vi "运维调试_氨氮总磷.vi"() -> ()   [LabVIEW 2016, in "氨氮总磷.lvlib"]
uses:
  <vilib>/Utility/miscctls.llb/LVPointTypeDef.ctl
  <vilib>/Utility/config.llb/NI_LVConfig.lvlib
panel:
  in  "氨氮自动测试量程配置":T1={"水样测试量程模式"=enum."AUTO", "空白核查量程模式"=enum."AUTO", "跨度核查量程模式"=enum."AUTO"}
  in  "总磷自动测试量程配置":T1={"水样测试量程模式"=enum."AUTO", "空白核查量程模式"=enum."AUTO", "跨度核查量程模式"=enum."AUTO"}
  in  "质控参数设置":bool
  out "字符串":string
  out "ADC":sgl
  out "温度2":sgl
  out "温度1":sgl
  out "总磷测量数据":T2(xcontrol)
  out "固件版本号":string
  in  "数组":string[](array[string])
  in  "备用系数写入":bool
  in  "备用系数读取":bool
  in  "备用系数":T3
  in  "量程切换阈值写入":bool
  in  "量程切换阈值读取":bool
  in  "量程切换阈值":cluster{"阈值":dbl, "标液浓度":dbl}
  in  "参数下拉列表":enum16{"氨氮", "总磷"}(ring)
  in  "量程下拉列表":enum16{"低量程", "高量程"}(ring)
  in  "测量模式下拉列表":enum16{"水样测量", "空白核查", "标样核查", "盲样测试", "加标回收"}(ring)
  in  "公式":cluster{"X^2":dbl, "X":dbl, "b":dbl}
  in  "写公式":bool
  in  "读公式":bool
  in  "精度":dbl=4.0
  in  "样品5 F0":dbl
  in  "样品5 F1":dbl
  in  "样品4 F1":dbl
  in  "样品4 F0":dbl
  in  "样品3 F0":dbl
  in  "样品3 F1":dbl
  in  "样品2 F0":dbl
  in  "样品2 F1":dbl
  in  "样品1 F1":dbl
  in  "样品1 F0":dbl
  in  "method":u16(ring) items=["最小二乘", "最小绝对残差", "Bisquare"]
  in  "模型":enum32{"线性", "多项式"}(ring)
  out "r^2":dbl format="%.7g"
  out "拟合公式":string
  in  "样品2启用":bool
  in  "样品5启用":bool
  in  "样品4启用":bool
  in  "样品3启用":bool
  in  "样品1启用":bool
  in  "标液浓度5":dbl
  in  "测量吸光度5":dbl
  in  "标液浓度4":dbl
  in  "测量吸光度4":dbl
  in  "标液浓度3":dbl
  in  "测量吸光度3":dbl
  in  "标液浓度2":dbl
  in  "测量吸光度2":dbl
  in  "测量吸光度1":dbl
  in  "标液浓度1":dbl
  out "XY图":cluster{"X Values":dbl[], "Y Values":dbl[]}[](graph)
  in  "返回":bool
  in  "设置":bool
  out "序列号":string="序列号"
  out "氨氮测量数据":T2(xcontrol)
  out "集成报警信息":string
  out "定时启动":bool
  out "总磷总氮运行状态":T4(xcontrol)
  in  "停止":bool
  in  "手动启动":bool
  in  "单步测试":bool
  in  "总磷氨氮调试":u16[](xcontrol)
  out "F3":sgl format="%#.6f"
  out "F2":sgl format="%#.6f"
  out "F1":sgl format="%#.6f"
  out "F0":sgl format="%#.6f"
  out "多列列表框":i32(listbox)
  # "参数设置"
  # "标液浓度"
  # "F0"
  # "F1"
  # "吸光值显示"
  # "样品一"
  # "辅\n助\n计\n算\n区"
  # "样品二"
  # "样品三"
  # "样品四"
  # "样品五"
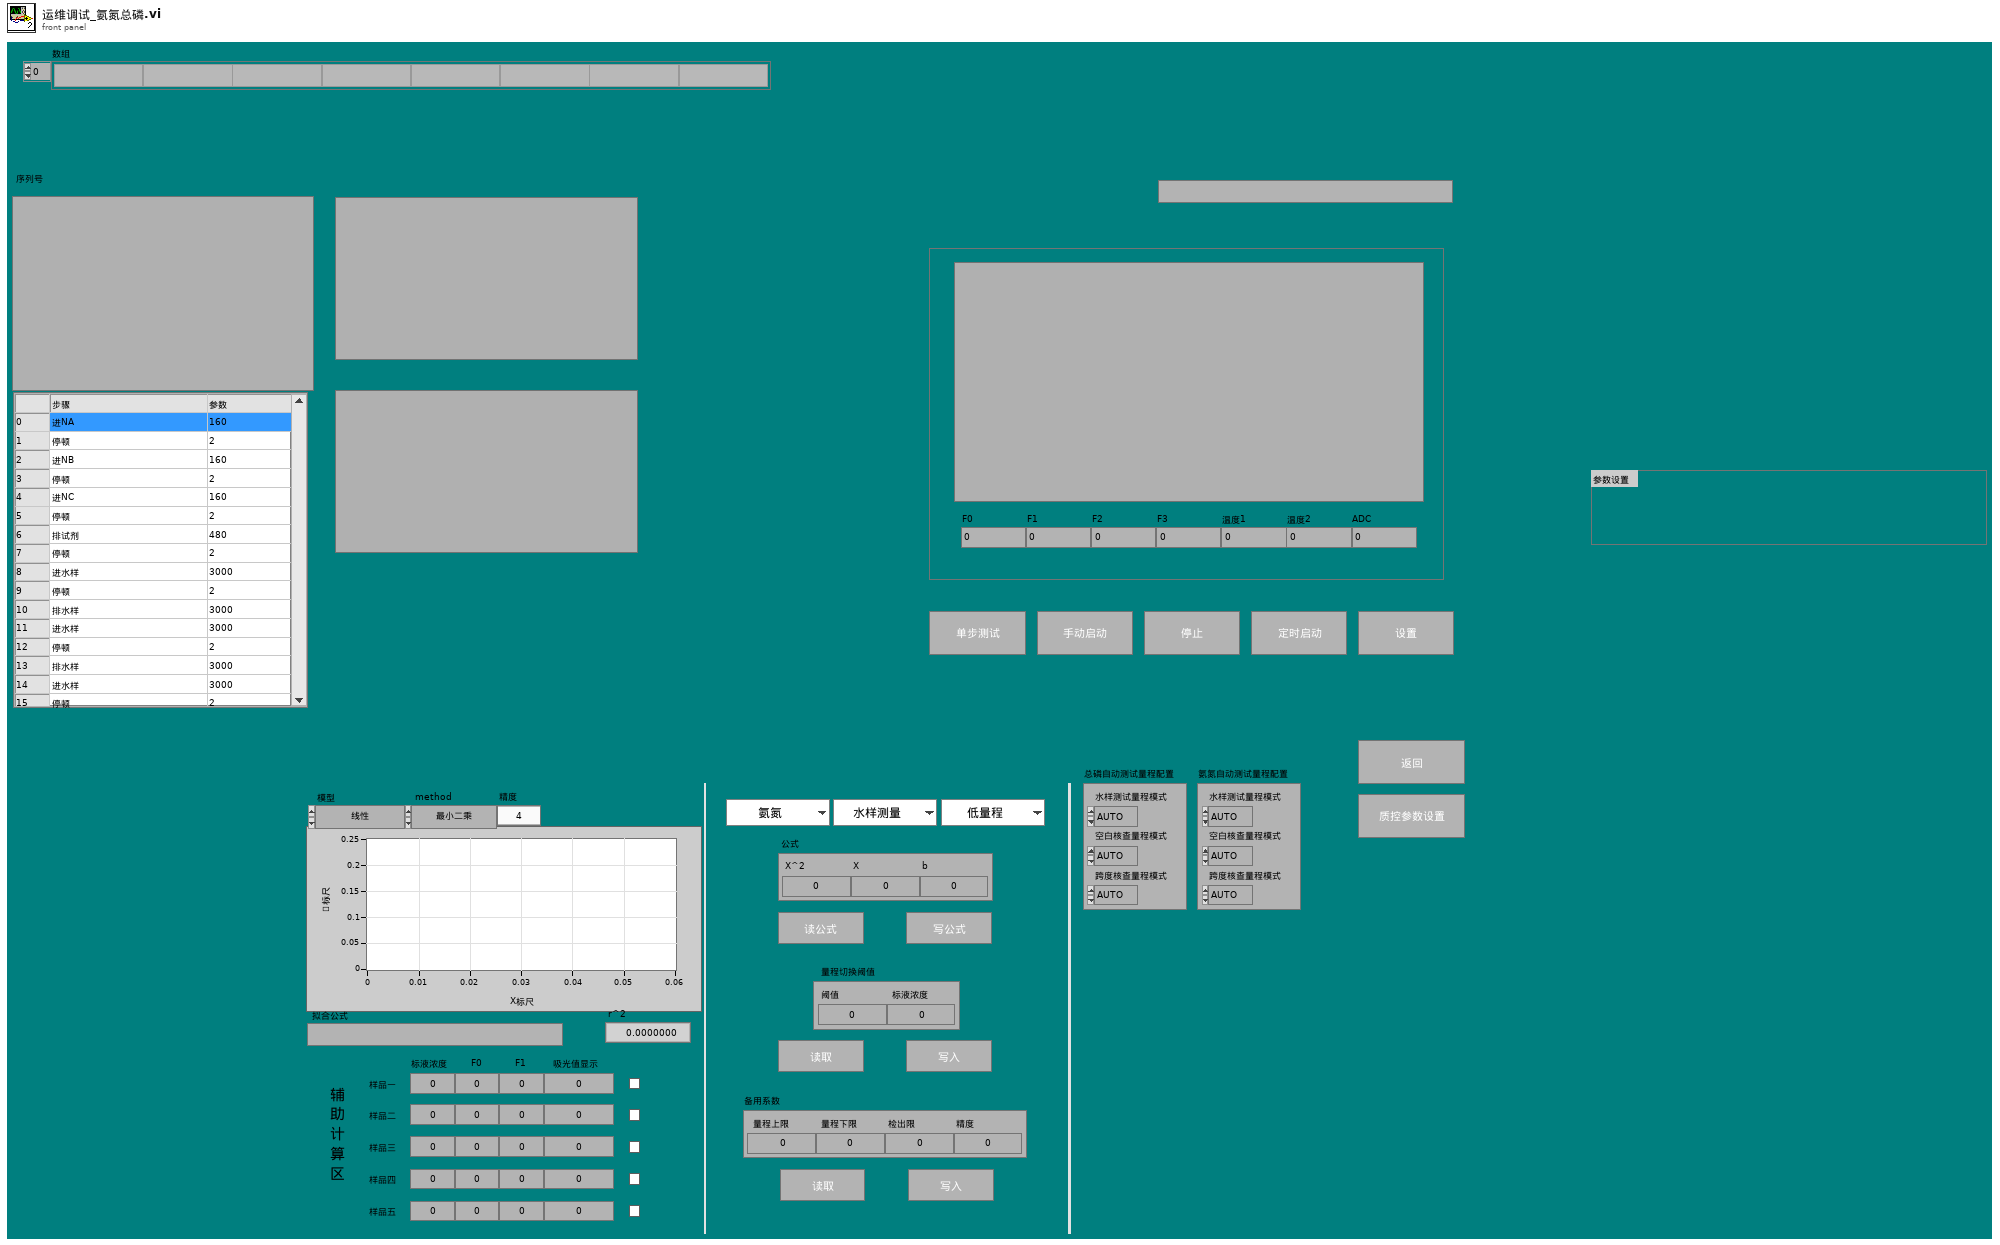
[diagram p1: front panel]
types:
  T1 = cluster{"水样测试量程模式":enum16{"H", "L", "AUTO"}, "空白核查量程模式":enum16{"H", "L", "AUTO"}, "跨度核查量程模式":enum16{"H", "L", "AUTO"}}
  T2 = cluster{"flowid":u16, "测量精度":u16, "测量数据区":cluster{"因子编码":u32, "单位":u16, "标样参考值":sgl, "水样数据时间":timestamp, "水样实测值":sgl, "水样数据标识":string, "标样数据时间":timestamp, "标样实测值":sgl, "标样数据标识":string, "空白数据时间":timestamp, "空白实测值":sgl, "空白数据标识":string, "零点核查数据时间":timestamp, "零点核查实测值":sgl, "零点核查数据标识":string, "跨度核查数据时间":timestamp, "跨度核查实测值":sgl, "跨度核查数据标识":string, "加标回收数据时间":timestamp, "加标回收实测值":sgl, "加标回收数据标识":string, "平行样数据时间":timestamp, "平行样实测值":sgl, "平行样数据标识":string}}
  T3 = cluster{"量程上限":dbl, "量程下限":dbl, "检出限":dbl, "精度":dbl}
  T4 = cluster{"系统时间":timestamp, "工作状态":enum16{"空闲", "水样测试", "标样核查", "零点核查", "跨度核查", "空白测试", "平行样测试", "加标回收", "空白校准", "标样校准", "初始化（清洗）"}, "测量模式":enum16{"待机", "连续模式", "周期模式", "定点模式", "受控模式", "手动模式"}, "告警代码":enum16{"无告警", "缺试剂告警", "缺水样告警", "缺蒸馏水告警", "缺标液告警", "仪表漏液告警", "标定异常告警", "超量程告警", "加热异常", "低试剂预警", "超上限告警", "超下限告警", "仪表内部其他异常", "滴定异常告警", "电极异常告警", "量程切换告警", "参数设置告警", "PH电极电位异常", "电导率电极异常", "浊度光度异常", "溶解氧电极异常", "溶解氧光强异常", "温度异常告警", "PH异常告警", "溶解氧异常告警", "电导率异常告警", "浊度异常告警", "叶绿素异常告警", "藻密度异常告警", "蓝绿藻异常告警", "ORP异常告警", "氨氮异常告警", "清洁刷异常告警", "SD卡异常告警", "蓝牙异常告警", "Wifi异常告警", "流程异常告警"}, "故障代码":enum16{"无故障", "电机故障", "温度故障", "通讯故障", "滴定故障"}, "日志代码":u16, "软件版本":u16, "F0":sgl, "F1":sgl, "F2":sgl, "F3":sgl, "T":sgl, "H":sgl, "id":u16, "flowid":u16, "量程":u16, "总磷控温温度1":sgl, "营养盐控温温度2":sgl, "ADC":sgl}
  T5 = cluster{"站号":u16, "量程切换":enum32{"H", "L", "AUTO"}, "控制命令":enum16{"启动测量", "标样核查", "零点核查", "跨度核查", "空白测试", "平行样测试", "加标回收", "空白校准", "标样校准", "初始化（清洗）", "停止测试", "仪器重启", "校时", "模式设置", "测量间隔设置"}, "模式设置":enum16{"待机", "连续模式", "周期模式", "定点模式", "受控模式", "手动模式"}, "测量间隔":u16}
  T6 = enum16{"启动测量", "标样核查", "零点核查", "跨度核查", "空白测试", "平行样测试", "加标回收", "空白校准", "标样校准", "初始化（清洗）", "停止测试", "仪器重启", "校时", "模式设置", "测量间隔设置"}
  T7 = cluster{"仪器测试类型":enum16{"水样测试", "标样核查", "空白测试", "跨度核查"}, "周期设置类型":enum16{"定点启动", "间隔启动"}, "定时功能启用":bool, "定时间隔":dbl, "24H周期设置":bool[]}
  T8 = enum32{"Bad", "Idle", "Run top level", "Running"}
  T9 = typedef "LVDateTimeRec.ctl" = cluster{"秒数的小数部分":dbl, "秒":i32, "分":i32, "时":i32, "日":i32, "月":i32, "年":i32, "天数（周）":i32, "天数（年）":i32, "DST":i32}
  T10 = typedef "LVPointTypeDef.ctl" = cluster{"Horizontal":i16, "Vertical":i16}
  T11 = cluster{"因子编码":u32, "单位":u16, "标样参考值":sgl, "水样数据时间":timestamp, "水样实测值":sgl, "水样数据标识":string, "标样数据时间":timestamp, "标样实测值":sgl, "标样数据标识":string, "空白数据时间":timestamp, "空白实测值":sgl, "空白数据标识":string, "零点核查数据时间":timestamp, "零点核查实测值":sgl, "零点核查数据标识":string, "跨度核查数据时间":timestamp, "跨度核查实测值":sgl, "跨度核查数据标识":string, "加标回收数据时间":timestamp, "加标回收实测值":sgl, "加标回收数据标识":string, "平行样数据时间":timestamp, "平行样实测值":sgl, "平行样数据标识":string}
  T12 = enum16{"空闲", "水样测试", "标样核查", "零点核查", "跨度核查", "空白测试", "平行样测试", "加标回收", "空白校准", "标样校准", "初始化（清洗）"}
  T13 = cluster{"启动模式":enum16{"标液测量", "水样测量", "零液测量", "盲样测量", "加标回收"}, "启动参数":u16, "量程":enum16{"低量程", "高量程"}}
  T14 = cluster{"时间标识":timestamp, "设备":string, "日志信息":string, "流程参数":string}
  T15 = cluster{"时间标识":timestamp, "设备":string, "日志信息":string}
  T16 = enum16{"无告警", "缺试剂告警", "缺水样告警", "缺蒸馏水告警", "缺标液告警", "仪表漏液告警", "标定异常告警", "超量程告警", "加热异常", "低试剂预警", "超上限告警", "超下限告警", "仪表内部其他异常", "滴定异常告警", "电极异常告警", "量程切换告警", "参数设置告警", "PH电极电位异常", "电导率电极异常", "浊度光度异常", "溶解氧电极异常", "溶解氧光强异常", "温度异常告警", "PH异常告警", "溶解氧异常告警", "电导率异常告警", "浊度异常告警", "叶绿素异常告警", "藻密度异常告警", "蓝绿藻异常告警", "ORP异常告警", "氨氮异常告警", "清洁刷异常告警", "SD卡异常告警", "蓝牙异常告警", "Wifi异常告警", "流程异常告警"}
  T17 = typedef "LVRowAndColumnUnsignedTypeDef.ctl" = cluster{"Row":u32, "Column":u32}
  T18 = typedef "NI_LVConfig.lvlib/Config Data RefNum.ctl" = refnum<k1>
  T19 = cluster{"XY图":cluster{"X Values":dbl[], "Y Values":dbl[]}[], "标液浓度1":dbl, "测量吸光度1":dbl, "测量吸光度2":dbl, "标液浓度2":dbl, "测量吸光度3":dbl, "标液浓度3":dbl, "测量吸光度4":dbl, "标液浓度4":dbl, "测量吸光度5":dbl, "标液浓度5":dbl, "样品1启用":bool, "样品3启用":bool, "样品4启用":bool, "样品5启用":bool, "样品2启用":bool, "拟合公式":string, "r^2":dbl, "模型":enum32{"线性", "多项式"}, "method":u16, "样品1 F0":dbl, "样品1 F1":dbl, "样品2 F1":dbl, "样品2 F0":dbl, "样品3 F1":dbl, "样品3 F0":dbl, "样品4 F0":dbl, "样品4 F1":dbl, "样品5 F1":dbl, "样品5 F0":dbl, "精度":dbl}
  T20 = cluster{"总磷跨度值":dbl, "总磷零点标准液浓度":dbl, "总磷跨度标准液浓度":dbl, "总磷标准液标准浓度":dbl, "氨氮跨度值":dbl, "氨氮零点标准液浓度":dbl, "氨氮跨度标准液浓度":dbl, "氨氮标准液标准浓度":dbl}
  T21 = cluster{"确定":bool, "总磷跨度值":dbl, "总磷零点标准液浓度":dbl, "总磷跨度标准液浓度":dbl, "总磷标准液标准浓度":dbl, "氨氮跨度值":dbl, "氨氮零点标准液浓度":dbl, "氨氮跨度标准液浓度":dbl, "氨氮标准液标准浓度":dbl}
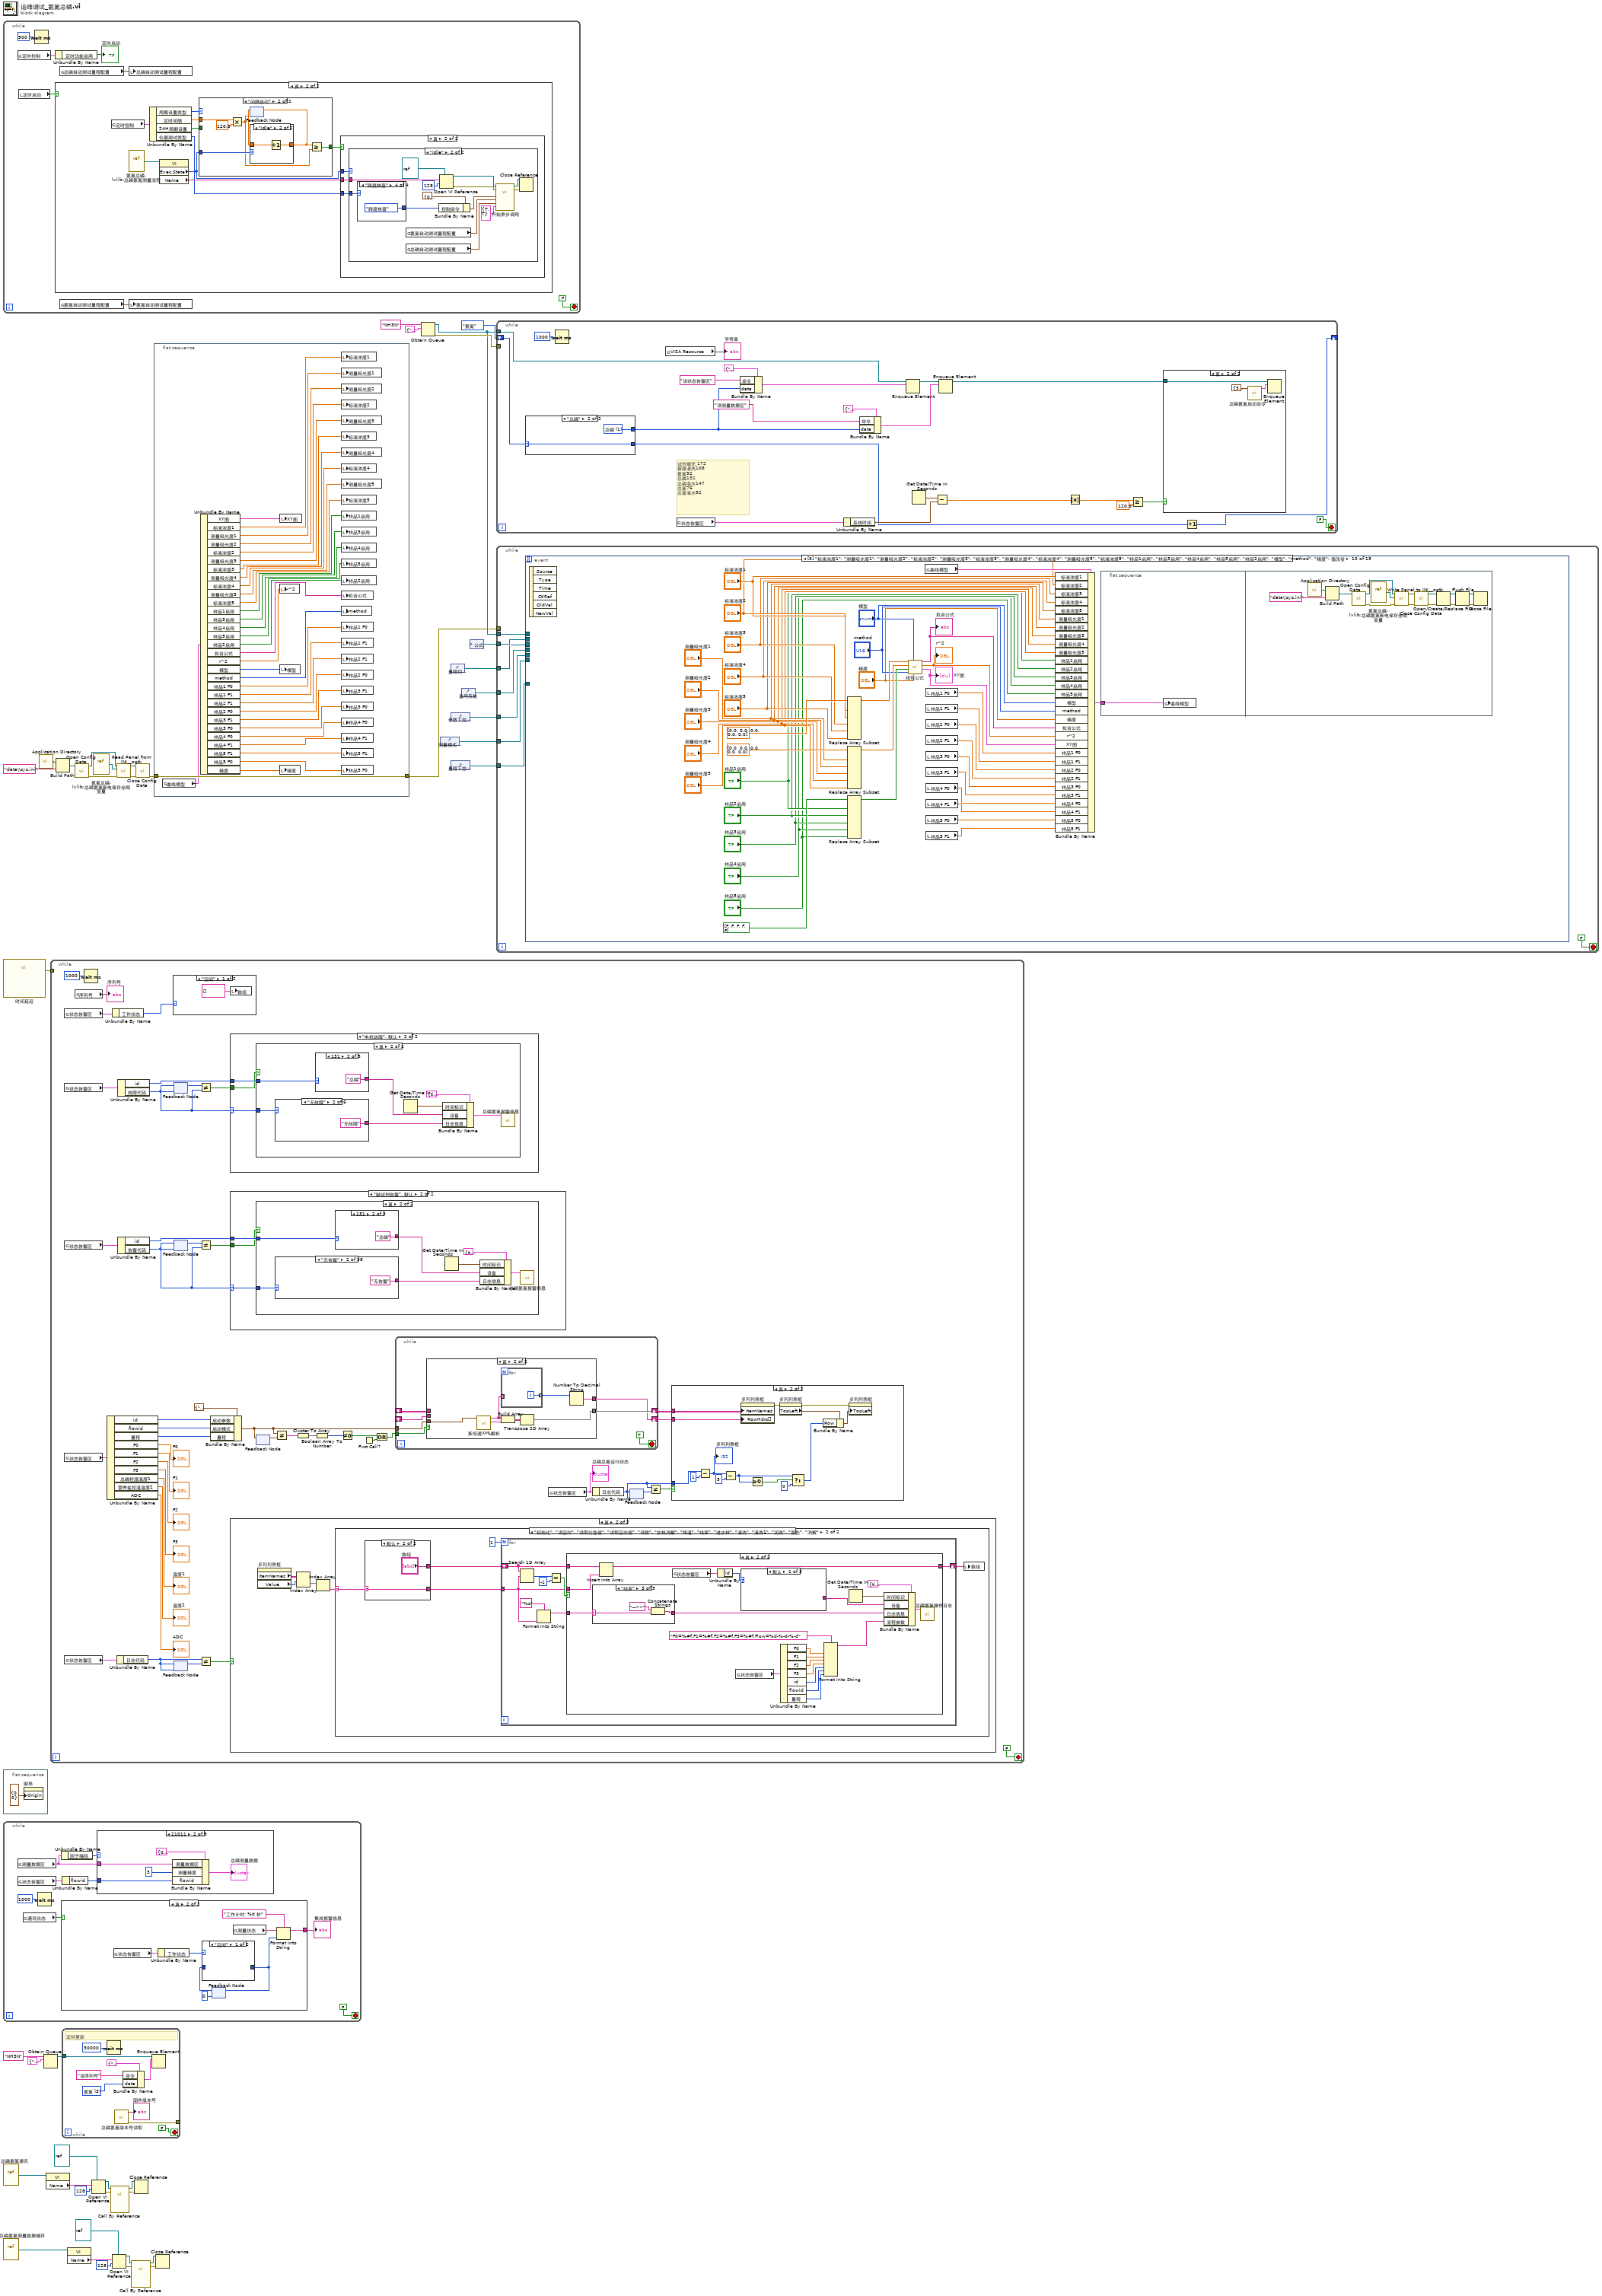
[diagram p0: block diagram]
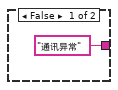
[diagram p2: hidden frame]
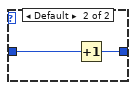
[diagram p3: hidden frame]
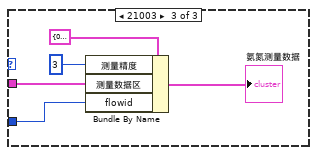
[diagram p5: hidden frame]
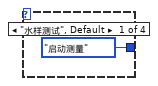
[diagram p9: hidden frame]
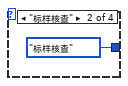
[diagram p10: hidden frame]
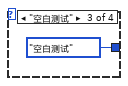
[diagram p11: hidden frame]
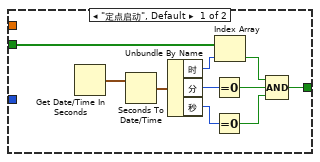
[diagram p12: hidden frame]
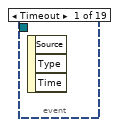
[diagram p14: hidden frame]
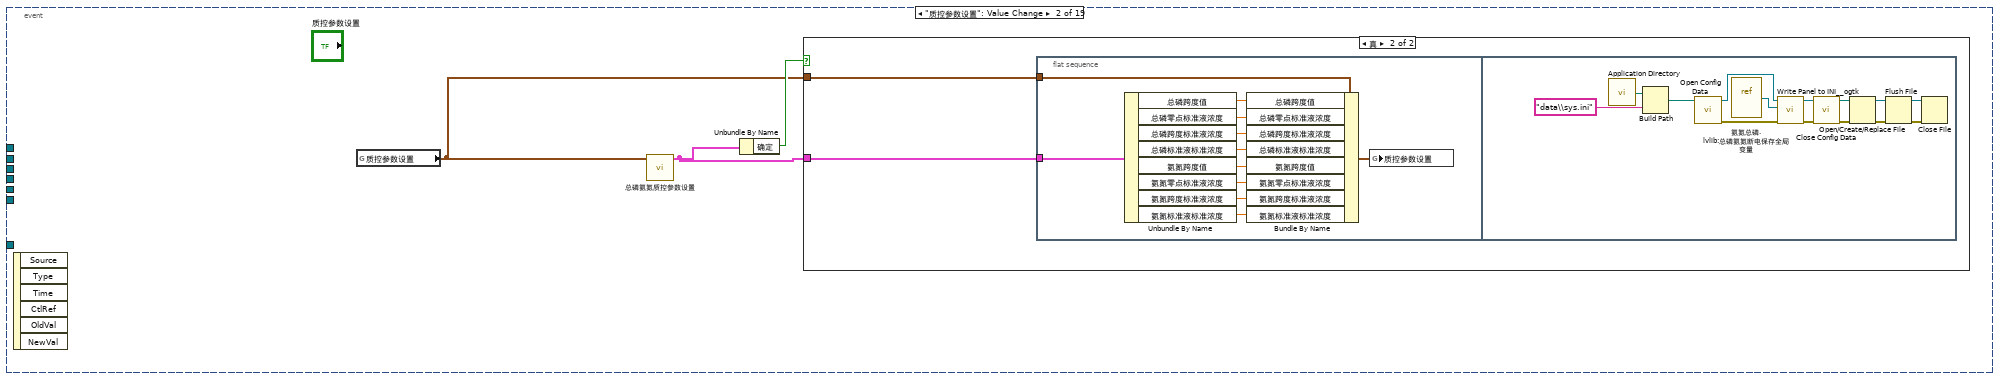
[diagram p15: hidden frame]
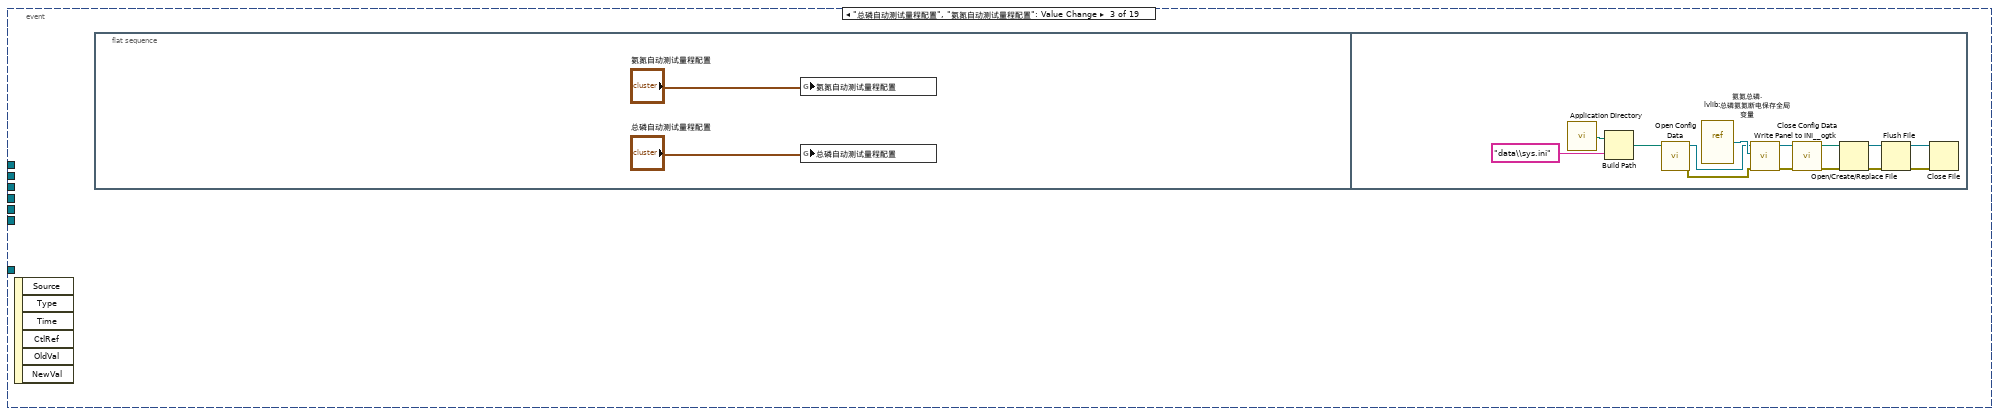
[diagram p17: hidden frame]
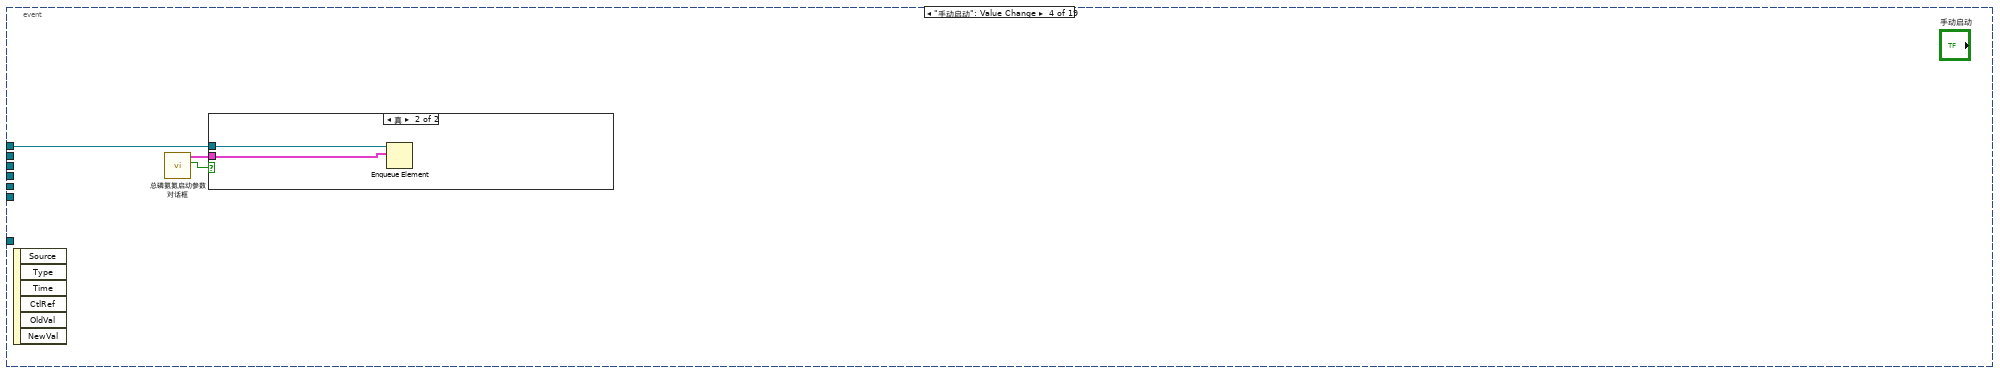
[diagram p18: hidden frame]
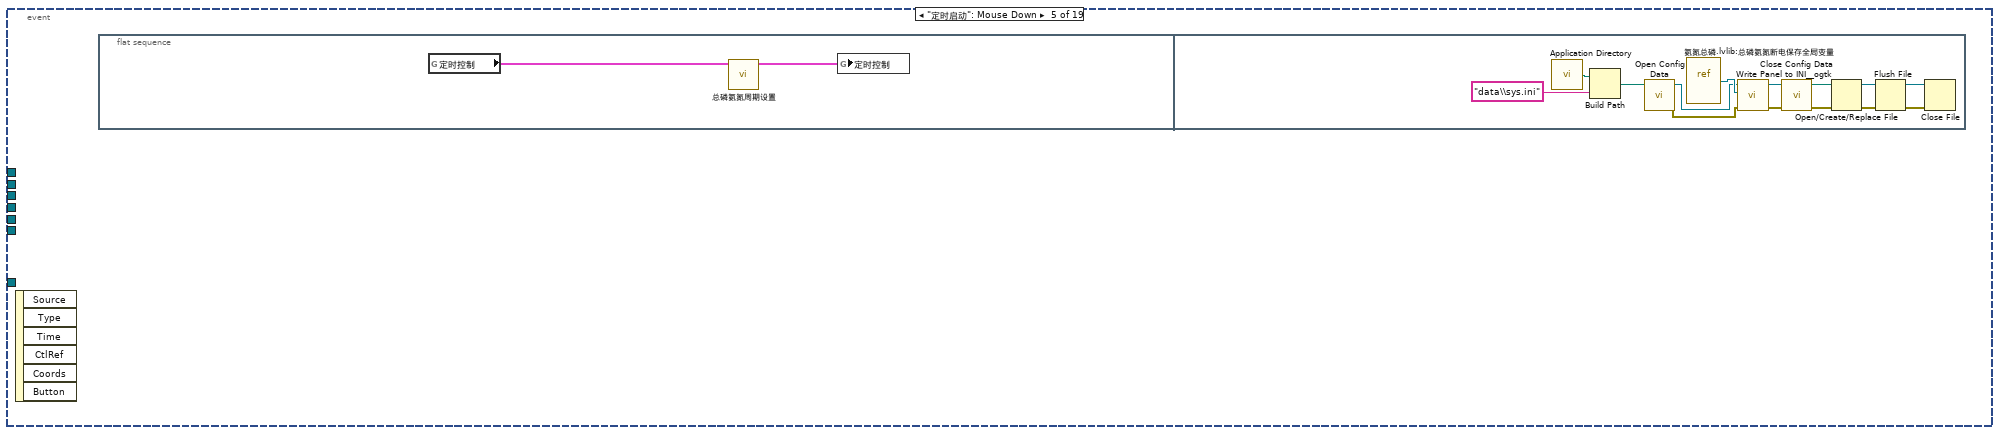
[diagram p20: hidden frame]
diagram:
  n1 = while {
    stop <- FALSE stop-if-true
    n2 = global read "总磷氨氮断电保存全局变量.vi" "定时控制"() -> (w46:T7)
    n3 = local read "定时启动"() -> (w42:bool)
    n4 = Wait (ms)(milliseconds to wait=u32 500 ("等待时间（毫秒）")) -> ()  [unwired: 1 out]
    n5 = Unbundle By Name(w46) -> ("定时功能启用"=→"定时启动":bool)
    n6 = case shown="真" w42 {
      frame False {
      }
      frame True {
        n7 = global read "总磷氨氮断电保存全局变量.vi" "定时控制"() -> (w49:T7)
        n8 = vi-ref "氨氮总磷.lvlib:总磷氨氮测量流程.vi"() -> (w53:refnum<vi>)
        n9 = Unbundle By Name(w49) -> ("周期设置类型"=w57:enum16{"定点启动", "间隔启动"}, "定时间隔"=w56:dbl, "24H周期设置"=w55:bool[], "仪器测试类型"=w52:enum16{"水样测试", "标样核查", "空白测试", "跨度核查"})
        n10 = property class="VI"(reference=w53) -> ("Exec.State"=w51:T8, "Name"=w50:string)  [unwired: 1 in, 2 out]
        n11 = case shown="\"间隔启动\"" w57 {
          tunnel: w56 -> [_ w92]
          tunnel: w55 -> [w88 _]
          tunnel: w51 -> [_ w95]
          tunnel: [w87 w90] -> w54
          frame "定点启动", Default {
            n12 = Get Date/Time In Seconds() -> (seconds since 1Jan1904=w86:timestamp)
            n13 = Seconds To Date/Time(time stamp (now)=w86) -> (date time rec=w85:T9)  [unwired: 1 in]
            n14 = Unbundle By Name(w85) -> ("时"=w84:i32, "分"=w82:i32, "秒"=w83:i32)
            n15 = Equal To 0?(x=w82) -> (x = 0?=w80:bool)
            n16 = Equal To 0?(x=w83) -> (x = 0?=w79:bool)
            n17 = Index Array(array=w88, index=w84) -> (element=w81:bool)
            n18 = Compound Arithmetic op=AND ("复合运算")(w81, w80, w79) -> (w87:bool)
          }
          frame "间隔启动" {
            n19 = Multiply(x=w92, y=120.0) -> (x*y=w89:dbl)
            n20 = feedback #1(w89) -> (w94:dbl)
            n21 = case shown="\"Idle\"" w95 {
              tunnel: w94 -> [_ w97]
              tunnel: [_ w96] -> w93
              frame "Bad", Default {
              }
              frame "Idle" {
                n22 = Increment(x=w97) -> (x+1=w96:dbl)
              }
            }
            n23 = feedback-in #1(w93) -> ()
            n24 = Greater Or Equal?(x=w93, y=w89) -> (x >= y?=w90:bool)
          }
        }
        n25 = case shown="真" w54 {
          tunnel: w50 -> [_ w60]
          tunnel: w52 -> [_ w59]
          tunnel: w51 -> [_ w58]
          frame False {
          }
          frame True {
            n26 = case shown="\"Idle\"" w58 {
              tunnel: w60 -> [_ w71]
              tunnel: w59 -> [_ w68]
              frame "Bad", Default {
              }
              frame "Idle" {
                n27 = case shown="\"跨度核查\"" w68 {
                  tunnel: [T6."启动测量" ("控制命令") T6."标样核查" ("控制命令") T6."空白测试" ("控制命令") T6."跨度核查" ("控制命令")] -> w67
                  frame "水样测试", Default {
                  }
                  frame "标样核查" {
                  }
                  frame "空白测试" {
                  }
                  frame "跨度核查" {
                  }
                }
                n28 = global read "总磷氨氮断电保存全局变量.vi" "氨氮自动测试量程配置"() -> (w64:T1)
                n29 = global read "总磷氨氮断电保存全局变量.vi" "总磷自动测试量程配置"() -> (w63:T1)
                n30 = Bundle By Name(cluster=T5 {"站号"=0, "量程切换"=enum."H", "控制命令"=enum."启动测量", "模式设置"=enum."待机", "测量间隔"=0} ("参数"), "控制命令"=w67) -> (w65:T5)
                n31 = Open VI Reference(type specifier VI Refnum (for type only)=refnum<vi> refnum, vi path=w71, options=128 ("选项")) -> (vi reference=w66:refnum<vi>, error out=w72:errorcluster)  [unwired: 3 in]
                n32 = call-by-ref "开始异步调用"(reference=w66, error in=w72, "启动参数"=cluster{"总磷":bool, "氨氮":bool} {"总磷"=TRUE, "氨氮"=TRUE}, "总磷量程模式"=w63, "氨氮量程模式"=w64, "参数"=w65) -> (reference out=w73:refnum<vi>, error out=w74:errorcluster)  [unwired: 8 in]
                n33 = Close Reference(reference=w73, error in (no error)=w74) -> ()  [unwired: 1 out]
              }
            }
          }
        }
      }
    }
    n34 = global read "总磷氨氮断电保存全局变量.vi" "总磷自动测试量程配置"() -> (w44:T1)
    n35 = global read "总磷氨氮断电保存全局变量.vi" "氨氮自动测试量程配置"() -> (w43:T1)
    n36 = local write "总磷自动测试量程配置"(w44) -> ()
    n37 = local write "氨氮自动测试量程配置"(w43) -> ()
  }
  n38 = call "时间延迟"() -> ("error out"=w14:errorcluster)  [unwired: 11 in]
  n39 = flat-sequence {
    frame #0 {
      n40 = property on="窗格" class="Pane"("Origin"=T10 {"Horizontal"=0, "Vertical"=0} ("原点")) -> ()  [unwired: 2 in, 2 out]
    }
  }
  n41 = while {
    stop <- FALSE stop-if-true
    n42 = global read "VAR总磷氨氮全局变量.vi" "测量数据区"() -> (w104:T11)
    n43 = global read "VAR总磷氨氮全局变量.vi" "状态告警区"() -> (w100:T4)
    n44 = global read "VAR总磷氨氮全局变量.vi" "通讯状态"() -> (w102:bool)
    n45 = Wait (ms)(milliseconds to wait=u32 1000 ("等待时间（毫秒）")) -> ()  [unwired: 1 out]
    n46 = Unbundle By Name(w104) -> ("因子编码"=w103:u32)
    n47 = case shown="真" w102 {
      tunnel: ["通讯异常" ("集成报警信息") w109] -> w101
      frame False {
      }
      frame True {
        n48 = global read "VAR总磷氨氮全局变量.vi" "状态告警区"() -> (w115:T4)
        n49 = Unbundle By Name(w115) -> ("工作状态"=w114:T12)
        n50 = feedback #2(0) -> (w112:i32)
        n51 = case shown="\"空闲\"" w114 {
          tunnel: w112 -> [_ w117]
          tunnel: [_ w116] -> w110
          frame "空闲" {
          }
          frame Default {
            n52 = Increment(x=w117) -> (x+1=w116:i32)
          }
        }
        n53 = feedback-in #2(w110) -> ()
        n54 = global read "VAR总磷氨氮全局变量.vi" "测量状态"() -> (w108:string)
        n55 = Format Into String(format string="工作计时: %d 秒" ("格式字符串"), initial string=w108, w110) -> (resulting string=w109:string)  [unwired: 1 in, 1 out]
      }
    }
    "集成报警信息" <- w101
    n56 = Unbundle By Name(w100) -> ("flowid"=w99:u16)
    n57 = case shown="21011" w103 {
      tunnel: w104 -> [_ w122 w127]
      tunnel: w99 -> [_ w120 w125]
      frame Default {
      }
      frame 21011 {
        n58 = Bundle By Name(cluster=T2 {"flowid"=0, "测量精度"=0, "测量数据区"={"因子编码"=0, "单位"=0, "标样参考值"=0.0, "水样数据时间"=timestamp(0 s since 1904-01-01), "水样实测值"=0.0, "水样数据标识"="", "标样数据时间"=timestamp(0 s since 1904-01-01), "标样实测值"=0.0, "标样数据标识"="", "空白数据时间"=timestamp(0 s since 1904-01-01), "空白实测值"=0.0, "空白数据标识"="", "零点核查数据时间"=timestamp(0 s since 1904-01-01), "零点核查实测值"=0.0, "零点核查数据标识"="", "跨度核查数据时间"=timestamp(0 s since 1904-01-01), "跨度核查实测值"=0.0, "跨度核查数据标识"="", "加标回收数据时间"=timestamp(0 s since 1904-01-01), "加标回收实测值"=0.0, "加标回收数据标识"="", "平行样数据时间"=timestamp(0 s since 1904-01-01), "平行样实测值"=0.0, "平行样数据标识"=""}} ("氨氮测量数据"), "测量数据区"=w122, "测量精度"=u16 3, "flowid"=w120) -> (→"总磷测量数据":T2)
      }
      frame 21003 {
        n59 = Bundle By Name(cluster=T2 {"flowid"=0, "测量精度"=0, "测量数据区"={"因子编码"=0, "单位"=0, "标样参考值"=0.0, "水样数据时间"=timestamp(0 s since 1904-01-01), "水样实测值"=0.0, "水样数据标识"="", "标样数据时间"=timestamp(0 s since 1904-01-01), "标样实测值"=0.0, "标样数据标识"="", "空白数据时间"=timestamp(0 s since 1904-01-01), "空白实测值"=0.0, "空白数据标识"="", "零点核查数据时间"=timestamp(0 s since 1904-01-01), "零点核查实测值"=0.0, "零点核查数据标识"="", "跨度核查数据时间"=timestamp(0 s since 1904-01-01), "跨度核查实测值"=0.0, "跨度核查数据标识"="", "加标回收数据时间"=timestamp(0 s since 1904-01-01), "加标回收实测值"=0.0, "加标回收数据标识"="", "平行样数据时间"=timestamp(0 s since 1904-01-01), "平行样实测值"=0.0, "平行样数据标识"=""}} ("氨氮测量数据"), "测量精度"=u16 3, "测量数据区"=w127, "flowid"=w125) -> (→"氨氮测量数据":T2)
      }
    }
  }
  n60 = vi-ref "总磷氨氮通讯.vi"() -> (w37:refnum<vi>)
  n61 = vi-ref "总磷氨氮测量数据储存.vi"() -> (w29:refnum<vi>)
  n62 = call <vilib>:"Application Directory.vi"() -> ("Application Directory"=w10:path)
  n63 = Obtain Queue(name (unnamed)="NH3N" ("名称（未命名）"), element data type=cluster{"命令":string, "data":variant} {"命令"="", "data"=variant}) -> (queue out=w11:refnum<queue>)  [unwired: 3 in, 2 out]
  n64 = property class="VI"(reference=w37) -> ("Name"=w36:string)  [unwired: 1 in, 2 out]
  n65 = while {
    tunnel: w14 -> [_]
    stop <- FALSE stop-if-true
    n66 = global read "VAR总磷氨氮全局变量.vi" "状态告警区"() -> (w136:T4)
    n67 = global read "VAR总磷氨氮全局变量.vi" "状态告警区"() -> (w142:T4)
    n68 = global read "VAR总磷氨氮全局变量.vi" "状态告警区"() -> (w147:T4)
    n69 = global read "VAR总磷氨氮全局变量.vi" "状态告警区"() -> (w159:T4)
    n70 = global read "VAR总磷氨氮全局变量.vi" "状态告警区"() -> (w133:T4)
    n71 = global read "VAR总磷氨氮全局变量.vi" "序列号"() -> (→"序列号":string)
    n72 = Wait (ms)(milliseconds to wait=u32 1000 ("等待时间（毫秒）")) -> ()  [unwired: 1 out]
    n73 = Unbundle By Name(w159) -> ("id"=w156:u16, "flowid"=w158:u16, "量程"=w157:u16, "F0"=→"F0":sgl, "F1"=→"F1":sgl, "F2"=→"F2":sgl, "F3"=→"F3":sgl, "总磷控温温度1"=→"温度1":sgl, "营养盐控温温度2"=→"温度2":sgl, "ADC"=→"ADC":sgl)
    n74 = Unbundle By Name(w136) -> ("工作状态"=w135:T12)
    n75 = Unbundle By Name(w133) -> ("日志代码"=w132:u16)
    n76 = Unbundle By Name(w142) -> ("id"=w141:u16, "故障代码"=w138:enum16{"无故障", "电机故障", "温度故障", "通讯故障", "滴定故障"})
    n77 = Unbundle By Name(w147) -> ("id"=w146:u16, "告警代码"=w143:T16)
    n78 = case shown="\"空闲\"" w135 {
      frame "空闲" {
        n79 = local write "数组"(string[] [] ("数组")) -> ()
      }
      frame "水样测试", Default {
      }
    }
    n80 = feedback #3(w138) -> (w139:enum16{"无故障", "电机故障", "温度故障", "通讯故障", "滴定故障"})
    n81 = feedback-in #3(w138) -> ()
    n82 = feedback #4(w143) -> (w144:T16)
    n83 = feedback-in #4(w143) -> ()
    n84 = feedback #5(w132) -> (w134:u16)
    n85 = feedback-in #5(w132) -> ()
    n86 = Not Equal?(x=w139, y=w138) -> (x != y?=w140:bool)
    n87 = Not Equal?(x=w144, y=w143) -> (x != y?=w145:bool)
    n88 = Not Equal?(x=w132, y=w134) -> (x != y?=w131:bool)
    n89 = Bundle By Name(cluster=T13 {"启动模式"=enum."加标回收", "启动参数"=1, "量程"=enum."低量程"} ("参数簇"), "启动参数"=w156, "启动模式"=w158, "量程"=w157) -> (w149:T13)
    n90 = case shown="\"电机故障\", 默认" w138 {
      selector: w138 -> [_ w227]
      tunnel: w141 -> [_ w228]
      tunnel: w140 -> [_ w226]
      frame "无故障" {
      }
      frame "电机故障", Default {
        n91 = case shown="真" w226 {
          tunnel: w228 -> [_ w235]
          tunnel: w227 -> [_ w230]
          frame False {
          }
          frame True {
            n92 = case shown="\"无故障\"" w230 {
              selector: w230 -> [w237 _ _ _ _ _]
              tunnel: [w236 "无故障" "电机故障" "温度故障" "通讯故障" "滴定故障"] -> w229
              frame Default {
                n93 = Format Into String(format string="%d" ("格式字符串"), initial string="未知" ("工作状态"), w237) -> (resulting string=w236:string)  [unwired: 1 in, 1 out]
              }
              frame "无故障" {
              }
              frame "电机故障" {
              }
              frame "温度故障" {
              }
              frame "通讯故障" {
              }
              frame "滴定故障" {
              }
            }
            n94 = case shown="131" w235 {
              tunnel: [_ "总磷" ("table输入") "氨氮" ("table输入")] -> w231
              frame Default {
              }
              frame 131 {
              }
              frame 92 {
              }
            }
            n95 = Get Date/Time In Seconds() -> (seconds since 1Jan1904=w232:timestamp)
            n96 = Bundle By Name(cluster=T15 {"时间标识"=timestamp(0 s since 1904-01-01), "设备"="", "日志信息"=""} ("data in"), "时间标识"=w232, "设备"=w231, "日志信息"=w229) -> (w233:T15)
            n97 = call "总磷氨氮报警信息.vi"("data in"=w233) -> ()  [unwired: 11 in]
          }
        }
      }
    }
    n98 = case shown="\"缺试剂告警\", 默认" w143 {
      selector: w143 -> [_ w248]
      tunnel: w146 -> [_ w249]
      tunnel: w145 -> [_ w247]
      frame "无告警" {
      }
      frame "缺试剂告警", Default {
        n99 = case shown="真" w247 {
          tunnel: w249 -> [_ w256]
          tunnel: w248 -> [_ w250]
          frame False {
          }
          frame True {
            n100 = case shown="\"无告警\"" w250 {
              selector: w250 -> [w258 _ _ _ _ _ _ _ _ _ _ _ _ _ _ _ _ _ _ _ _ _ _ _ _ _ _ _ _ _ _ _ _ _ _ _ _ _]
              tunnel: [w257 "无告警" "缺试剂告警" "缺水样告警" "缺蒸馏水告警" "缺标液告警" "仪表漏液告警" "标定异常告警" "超量程告警" "加热异常" "低试剂预警" "超上限告警" "超下限告警" "仪表内部其他异常" "滴定异常告警" "电极异常告警" "量程切换告警" "参数设置告警" "PH电极电位异常" "电导率电极异常" "浊度光度异常" "溶解氧电极异常" "溶解氧光强异常" "温度异常告警" "PH异常告警" "溶解氧异常告警" "电导率异常告警" "浊度异常告警" "叶绿素异常告警" "藻密度异常告警" "蓝绿藻异常告警" "ORP异常告警" "氨氮异常告警" "清洁刷异常告警" "SD卡异常告警" "蓝牙异常告警" "WiFi异常告警" "流程异常告警"] -> w251
              frame Default {
                n101 = Format Into String(format string="%d" ("格式字符串"), initial string="未知" ("工作状态"), w258) -> (resulting string=w257:string)  [unwired: 1 in, 1 out]
              }
              frame "无告警" {
              }
              frame "缺试剂告警" {
              }
              frame "缺水样告警" {
              }
              frame "缺蒸馏水告警" {
              }
              frame "缺标液告警" {
              }
              frame "仪表漏液告警" {
              }
              frame "标定异常告警" {
              }
              frame "超量程告警" {
              }
              frame "加热异常" {
              }
              frame "低试剂预警" {
              }
              frame "超上限告警" {
              }
              frame "超下限告警" {
              }
              frame "仪表内部其他异常" {
              }
              frame "滴定异常告警" {
              }
              frame "电极异常告警" {
              }
              frame "量程切换告警" {
              }
              frame "参数设置告警" {
              }
              frame "PH电极电位异常" {
              }
              frame "电导率电极异常" {
              }
              frame "浊度光度异常" {
              }
              frame "溶解氧电极异常" {
              }
              frame "溶解氧光强异常" {
              }
              frame "温度异常告警" {
              }
              frame "PH异常告警" {
              }
              frame "溶解氧异常告警" {
              }
              frame "电导率异常告警" {
              }
              frame "浊度异常告警" {
              }
              frame "叶绿素异常告警" {
              }
              frame "藻密度异常告警" {
              }
              frame "蓝绿藻异常告警" {
              }
              frame "ORP异常告警" {
              }
              frame "氨氮异常告警" {
              }
              frame "清洁刷异常告警" {
              }
              frame "SD卡异常告警" {
              }
              frame "蓝牙异常告警" {
              }
              frame "Wifi异常告警" {
              }
              frame "流程异常告警" {
              }
            }
            n102 = case shown="131" w256 {
              tunnel: [_ "总磷" ("table输入") "氨氮" ("table输入")] -> w252
              frame Default {
              }
              frame 131 {
              }
              frame 92 {
              }
            }
            n103 = Get Date/Time In Seconds() -> (seconds since 1Jan1904=w253:timestamp)
            n104 = Bundle By Name(cluster=T15 {"时间标识"=timestamp(0 s since 1904-01-01), "设备"="", "日志信息"=""} ("data in"), "时间标识"=w253, "设备"=w252, "日志信息"=w251) -> (w254:T15)
            n105 = call "总磷氨氮报警信息.vi"("data in"=w254) -> ()  [unwired: 11 in]
          }
        }
      }
    }
    n106 = case shown="真" w131 {
      frame False {
      }
      frame True {
        n107 = property on="多列列表框" class="MCListbox (严格)"() -> ("ItemNames"=w176:string[][], "Value"=w177:i32)  [unwired: 2 in, 2 out]
        n108 = Index Array(array=w176, index (row)=w177) -> (element=w175:string[])  [unwired: 1 in]
        n109 = Index Array(array=w175) -> (element=w174:string)  [unwired: 1 in]
        n110 = case shown="\"初始化\", \"读空白\", \"读取比色值\", \"读取空白值\", \"读数\", \"加热消解\", \"降温\", \"结束\", \"进水样\", \"清洗\", \"清洗1\", \"润洗\", \"显色\", \"消解\"" w174 {
          selector: w174 -> [_ w180]
          frame Default {
          }
          frame "初始化", "读空白", "读取比色值", "读取空白值", "读数", "加热消解", "降温", "结束", "进水样", "清洗", "清洗1", "润洗", "显色", "消解" {
            n111 = case shown="默认" w180 {
              selector: w180 -> [w184 w186]
              tunnel: [w184 w186] -> w179
              tunnel: [string[] [] ("数组") "数组"] -> w178
              frame "读数" {
              }
              frame Default {
              }
            }
            n112 = for {
              N: 1 -> [_]
              tunnel: w179 -> [w188]
              shift-right: [w187] -> w181
              shift-left: w178 -> [w189]
              n113 = Search 1D Array(1D array=w189, element=w188) -> (index of element=w192:i32)  [unwired: 1 in]
              n114 = Format Into String(format string="%s" ("格式字符串"), w188) -> (resulting string=w193:string)  [unwired: 2 in, 1 out]
              n115 = Equal?(x=w192, y=-1) -> (x = y?=w190:bool)
              n116 = case shown="真" w190 {
                tunnel: w193 -> [_ w197]
                tunnel: w189 -> [w195 w201]
                tunnel: w188 -> [_ w200]
                tunnel: [w195 w199] -> w187
                frame False {
                }
                frame True {
                  n117 = case shown="\"结束\"" w197 {
                    selector: w197 -> [w217 w220 w223]
                    tunnel: [w217 w219 w222] -> w196
                    frame Default {
                    }
                    frame "初始化" {
                      n118 = Concatenate Strings("-->>" ("字符串"), w220) -> (w219:string)
                    }
                    frame "结束" {
                      n119 = Concatenate Strings("-->>" ("字符串"), w223) -> (w222:string)
                    }
                  }
                  n120 = Insert Into Array(array=w201, new element=w200) -> (w199:string[])  [unwired: 1 in]
                  n121 = global read "VAR总磷氨氮全局变量.vi" "状态告警区"() -> (w216:T4)
                  n122 = Unbundle By Name(w216) -> ("id"=w215:u16)
                  n123 = global read "VAR总磷氨氮全局变量.vi" "状态告警区"() -> (w211:T4)
                  n124 = case shown="默认" w215 {
                    tunnel: [_ "总磷" ("table输入") "氨氮" ("table输入")] -> w213
                    frame Default {
                    }
                    frame 131 {
                    }
                    frame 92 {
                    }
                  }
                  n125 = Unbundle By Name(w211) -> ("F0"=w208:sgl, "F1"=w207:sgl, "F2"=w206:sgl, "F3"=w205:sgl, "id"=w204:u16, "flowid"=w203:u16, "量程"=w202:u16)
                  n126 = Format Into String(format string="F0=%#f,F1=%#f,F2=%#f,F3=%#f,Flow=%d-%-d-%-d" ("格式字符串"), w208, w207, w206, w205, w204, w203, w202) -> (resulting string=w209:string)  [unwired: 2 in, 1 out]
                  n127 = Get Date/Time In Seconds() -> (seconds since 1Jan1904=w212:timestamp)
                  n128 = Bundle By Name(cluster=T14 {"时间标识"=timestamp(0 s since 1904-01-01), "设备"="", "日志信息"="", "流程参数"=""} ("data in"), "时间标识"=w212, "设备"=w213, "日志信息"=w196, "流程参数"=w209) -> (w214:T14)
                  n129 = call "总磷氨氮操作日志.vi"("data in"=w214) -> ()  [unwired: 11 in]
                }
              }
            }
            n130 = local write "数组"(w181) -> ()
          }
        }
      }
    }
    n131 = feedback #6() -> (w165:T13)  [unwired: 1 in]
    n132 = feedback-in #6(w149) -> ()
    n133 = Not Equal?(x=w149, y=w165) -> (x != y?=w166:cluster{"启动模式":bool, "启动参数":bool, "量程":bool})
    n134 = Cluster To Array(cluster=w166) -> (array=w167:bool[])
    n135 = Boolean Array To Number(Boolean array=w167) -> (number=w168:u32)
    n136 = Not Equal To 0?(x=w168) -> (x != 0?=w161:bool)
    n137 = First Call?() -> (First Call?: T/F=w162:bool)
    n138 = Or(x=w161, y=w162) -> (x .or. y?=w160:bool)
    n139 = while {
      tunnel: w160 -> [w306]
      tunnel: w149 -> [w305]
      shift-right: [w304] -> w164
      shift-left: _ -> [w300]
      shift-right: [w303] -> w163
      shift-left: _ -> [w301]
      stop <- TRUE stop-if-true
      n140 = case shown="真" w306 {
        tunnel: [w308 w315] -> w303
        tunnel: [w307 w314] -> w304
        tunnel: w305 -> [_ w309]
        tunnel: w301 -> [w308 _]
        tunnel: w300 -> [w307 _]
        frame False {
        }
        frame True {
          n141 = call "斯坦道XML解析.vi"("参数簇"=w309) -> ("步骤时间"=w310:string[], "步骤名"=w312:string[])  [unwired: 9 in]
          n142 = for {
            tunnel: w312 -> [_] mode=indexing
            tunnel: [w316] -> w313 mode=indexing
            i -> [w316]
          }
          n143 = Build Array(w312, w310) -> (w311:string[][])
          n144 = Transpose 2D Array(2D array=w311) -> (transposed array=w314:string[][])
          n145 = Number To Decimal String(number=w313) -> (decimal integer string=w315:string[])  [unwired: 1 in]
        }
      }
    }
    n146 = global read "VAR总磷氨氮全局变量.vi" "状态告警区"() -> (w150:T4)
    "总磷总氮运行状态" <- w150
    n147 = Unbundle By Name(w150) -> ("日志代码"=w137:u16)
    n148 = feedback-in #7(w137) -> ()
    n149 = feedback #7(w137) -> (w170:u16)
    n150 = Not Equal?(x=w137, y=w170) -> (x != y?=w169:bool)
    n151 = case shown="真" w169 {
      tunnel: w137 -> [_ w319]
      tunnel: w164 -> [_ w326]
      tunnel: w163 -> [_ w325]
      frame False {
      }
      frame True {
        n152 = Subtract(x=w319, y=1) -> (x-y=w317:i32)
        "多列列表框" <- w317
        n153 = Subtract(x=w317, y=5) -> (x-y=w321:i32)
        n154 = property on="多列列表框" class="MCListbox (严格)"("ItemNames"=w326, "RowHdrs[]"=w325) -> (error out=w327:errorcluster)  [unwired: 2 in, 1 out]
        n155 = Greater Or Equal To 0?(x=w321) -> (x >= 0?=w320:bool)
        n156 = property on="多列列表框" class="MCListbox (严格)"(error in=w327) -> (error out=w328:errorcluster, "TopLeft"=w329:T17)  [unwired: 1 in, 1 out]
        n157 = Select(t=w321, s=w320, f=0) -> (s? t:f=w322:i32)
        n158 = Bundle By Name(cluster=w329, "Row"=w322) -> (w330:T17)
        n159 = property on="多列列表框" class="MCListbox (严格)"(error in=w328, "TopLeft"=w330) -> ()  [unwired: 1 in, 2 out]
      }
    }
  }
  n160 = Build Path(base path=w10, name or relative path="data\\sys.ini" ("名称或相对路径")) -> (appended path=w8:path)
  n161 = while {
    tunnel: w11 -> [w335]
    tunnel: [w332] -> _
    stop <- FALSE stop-if-true
    w336 = u16 3 items=["总磷"=1, "氨氮"=3] ("站号")
    # "定时更新"
    n162 = Wait (ms)(milliseconds to wait=u32 30000 ("等待时间（毫秒）")) -> ()  [unwired: 1 out]
    n163 = call "总磷氨氮版本号读取.vi"() -> ("error out"=w332:errorcluster, "固件版本号"=→"固件版本号":string)  [unwired: 10 in]
    n164 = Bundle By Name(cluster=cluster{"命令":string, "data":variant} {"命令"="", "data"=variant} ("元素"), "命令"="读序列号", "data"=w336) -> (w334:cluster{"命令":string, "data":variant})
    n165 = Enqueue Element(queue=w335, element=w334) -> ()  [unwired: 2 in, 3 out]
  }
  n166 = property class="VI"(reference=w29) -> ("Name"=w22:string)  [unwired: 1 in, 2 out]
  n167 = call <vilib>:"Open Config Data.vi"("configuration file path"=w8) -> ("error out"=w4:errorcluster, "refnum"=w7:T18)  [unwired: 8 in, 1 out]
  n168 = Open VI Reference(type specifier VI Refnum (for type only)=refnum<vi> refnum, vi path=w36, options=128 ("选项")) -> (vi reference=w34:refnum<vi>, error out=w32:errorcluster)  [unwired: 3 in]
  n169 = vi-ref "氨氮总磷.lvlib:总磷氨氮断电保存全局变量.vi"() -> (w6:refnum<vi>)
  n170 = call-by-ref "?"(reference=w34, error in=w32) -> (reference out=w30:refnum<vi>, error out=w31:errorcluster)  [unwired: 12 in]
  n171 = Open VI Reference(type specifier VI Refnum (for type only)=refnum<vi> refnum, vi path=w22, options=128 ("选项")) -> (vi reference=w24:refnum<vi>, error out=w26:errorcluster)  [unwired: 3 in]
  n172 = call <userlib>:"Read Panel from INI__ogtk.vi"("error in (no error)"=w4, "VI ref"=w6, "refnum"=w7) -> ("error out"=w3:errorcluster, "refnum out"=w5:T18)  [unwired: 7 in]
  n173 = call-by-ref "?"(reference=w24, error in=w26) -> (reference out=w28:refnum<vi>, error out=w27:errorcluster)  [unwired: 12 in]
  n174 = Close Reference(reference=w30, error in (no error)=w31) -> ()  [unwired: 1 out]
  n175 = call <vilib>:"Close Config Data.vi"("error in (no error)"=w3, "refnum"=w5) -> ("error out"=w2:errorcluster)  [unwired: 8 in, 1 out]
  n176 = flat-sequence {
    tunnel: w2 -> [w372]
    tunnel: [w372] -> w1
    frame #0 {
      n177 = global read "总磷氨氮断电保存全局变量.vi" "曲线模型"() -> (w371:T19)
      n178 = Unbundle By Name(w371) -> ("XY图"=w370:cluster{"X Values":dbl[], "Y Values":dbl[]}[], "标液浓度1"=w369:dbl, "测量吸光度1"=w368:dbl, "测量吸光度2"=w367:dbl, "标液浓度2"=w366:dbl, "测量吸光度3"=w365:dbl, "标液浓度3"=w364:dbl, "测量吸光度4"=w363:dbl, "标液浓度4"=w362:dbl, "测量吸光度5"=w361:dbl, "标液浓度5"=w360:dbl, "样品1启用"=w359:bool, "样品3启用"=w357:bool, "样品4启用"=w356:bool, "样品5启用"=w355:bool, "样品2启用"=w358:bool, "拟合公式"=w354:string, "r^2"=w353:dbl, "模型"=w352:enum32{"线性", "多项式"}, "method"=w351:u16, "样品1 F0"=w349:dbl, "样品1 F1"=w348:dbl, "样品2 F1"=w347:dbl, "样品2 F0"=w346:dbl, "样品3 F1"=w345:dbl, "样品3 F0"=w344:dbl, "样品4 F0"=w343:dbl, "样品4 F1"=w342:dbl, "样品5 F1"=w340:dbl, "样品5 F0"=w341:dbl, "精度"=w350:dbl)
      n179 = local write "XY图"(w370) -> ()
      n180 = local write "r^2"(w353) -> ()
      n181 = local write "模型"(w352) -> ()
      n182 = local write "精度"(w350) -> ()
      n183 = local write "标液浓度1"(w369) -> ()
      n184 = local write "测量吸光度1"(w368) -> ()
      n185 = local write "测量吸光度2"(w367) -> ()
      n186 = local write "标液浓度2"(w366) -> ()
      n187 = local write "测量吸光度3"(w365) -> ()
      n188 = local write "标液浓度3"(w364) -> ()
      n189 = local write "测量吸光度4"(w363) -> ()
      n190 = local write "标液浓度4"(w362) -> ()
      n191 = local write "测量吸光度5"(w361) -> ()
      n192 = local write "标液浓度5"(w360) -> ()
      n193 = local write "样品1启用"(w359) -> ()
      n194 = local write "样品3启用"(w357) -> ()
      n195 = local write "样品4启用"(w356) -> ()
      n196 = local write "样品5启用"(w355) -> ()
      n197 = local write "样品2启用"(w358) -> ()
      n198 = local write "拟合公式"(w354) -> ()
      n199 = local write "method"(w351) -> ()
      n200 = local write "样品1 F0"(w349) -> ()
      n201 = local write "样品1 F1"(w348) -> ()
      n202 = local write "样品2 F1"(w347) -> ()
      n203 = local write "样品2 F0"(w346) -> ()
      n204 = local write "样品3 F1"(w345) -> ()
      n205 = local write "样品3 F0"(w344) -> ()
      n206 = local write "样品4 F0"(w343) -> ()
      n207 = local write "样品4 F1"(w342) -> ()
      n208 = local write "样品5 F1"(w340) -> ()
      n209 = local write "样品5 F0"(w341) -> ()
    }
  }
  n210 = Close Reference(reference=w28, error in (no error)=w27) -> ()  [unwired: 1 out]
  n211 = Obtain Queue(name (unnamed)="NH3N" ("名称（未命名）"), element data type=cluster{"命令":string, "data":variant} {"命令"="", "data"=variant}) -> (queue out=w38:refnum<queue>, error out=w39:errorcluster)  [unwired: 3 in, 1 out]
  n212 = control-ref of="测量模式下拉列表"() -> (w18:refnum<vi>)
  n213 = control-ref of="量程切换阈值"() -> (w16:refnum<vi>)
  n214 = control-ref of="参数下拉列表"() -> (w19:refnum<vi>)
  n215 = control-ref of="量程下拉列表"() -> (w20:refnum<vi>)
  n216 = control-ref of="备用系数"() -> (w15:refnum<vi>)
  n217 = control-ref of="公式"() -> (w17:refnum<vi>)
  n218 = while {
    tunnel: w38 -> [w390]
    tunnel: w39 -> [_]
    shift-right: [w385] -> _
    shift-left: enum16{"氨氮", "总磷"}."氨氮" ("枚举") -> [w376]
    stop <- FALSE stop-if-true
    # "试剂填充 172 \n管路清洗108\n氨氮92\n总磷131\n总磷海水147\n总氮76\n总氮海水92"
    n219 = case shown="\"总磷\"" w376 {
      selector: w376 -> [w396 w399]
      tunnel: [w397 w398] -> w375
      tunnel: [w396 w399] -> w374
      frame "氨氮", Default {
        w397 = u16 3 items=["总磷"=1, "氨氮"=3] ("站号")
      }
      frame "总磷" {
        w398 = u16 1 items=["总磷"=1, "氨氮"=3] ("站号")
      }
    }
    n220 = Wait (ms)(milliseconds to wait=u32 1000 ("等待时间（毫秒）")) -> ()  [unwired: 1 out]
    n221 = global read "VAR总磷氨氮全局变量.vi" "VISA Resource"() -> (→"字符串":refnum<visa-resource-name>)
    n222 = global read "VAR总磷氨氮全局变量.vi" "状态告警区"() -> (w383:T4)
    n223 = Bundle By Name(cluster=cluster{"命令":string, "data":variant} {"命令"="", "data"=variant} ("元素"), "命令"="读状态告警区", "data"=w375) -> (w392:cluster{"命令":string, "data":variant})
    n224 = Unbundle By Name(w383) -> ("系统时间"=w382:timestamp)
    n225 = Bundle By Name(cluster=cluster{"命令":string, "data":variant} {"命令"="", "data"=variant} ("元素"), "命令"="读测量数据区", "data"=w375) -> (w388:cluster{"命令":string, "data":variant})
    n226 = Enqueue Element(queue=w390, element=w392) -> (queue out=w386:refnum<queue>)  [unwired: 2 in, 2 out]
    n227 = Get Date/Time In Seconds() -> (seconds since 1Jan1904=w381:timestamp)
    n228 = Subtract(x=w381, y=w382) -> (x-y=w380:dbl)
    n229 = Enqueue Element(queue=w386, element=w388) -> (queue out=w384:refnum<queue>)  [unwired: 2 in, 2 out]
    n230 = Absolute Value(x=w380) -> (abs(x)=w379:dbl)
    n231 = Greater Or Equal?(x=w379, y=120.0) -> (x >= y?=w377:bool)
    n232 = case shown="真" w377 {
      tunnel: w384 -> [_ w401]
      frame False {
      }
      frame True {
        n233 = call "总磷氨氮启动命令.vi"("参数"=T5 {"站号"=3, "量程切换"=enum."AUTO", "控制命令"=enum."校时", "模式设置"=enum."待机", "测量间隔"=0}) -> ("启动命令"=w400:cluster{"命令":string, "data":variant})  [unwired: 10 in]
        n234 = Enqueue Element(queue=w401, element=w400) -> ()  [unwired: 2 in, 3 out]
      }
    }
    n235 = Increment(x=w374) -> (x+1=w385:enum16{"氨氮", "总磷"})
  }
  n236 = while {
    tunnel: w38 -> [w409]
    tunnel: w20 -> [w408]
    tunnel: w19 -> [w407]
    tunnel: w18 -> [w406]
    tunnel: w17 -> [w405]
    tunnel: w16 -> [w404]
    tunnel: w15 -> [w403]
    tunnel: w1 -> [_]
    stop <- FALSE stop-if-true
    n237 = event shown="[9] \"标液浓度1\", \"测量吸光度1\", \"测量吸光度2\", \"标液浓度2\", \"测量吸光度3\", \"标液浓度3\", \"测量吸光度4\", \"标液浓度4\", \"测量吸光度5\", \"标液浓度5\", \"样品1启用\", \"样品3启用\", \"样品4启用\", \"样品5启用\", \"样品2启用\", \"模型\", \"method\", \"精度\": 值改变" {
      selector: _ -> [_ _ _ _ _ _ _ _ _ _ _ _ _ _ _ _ _ _ _]
      dyn-events: _ -> [_ _ _ _ _ _ _ _ _ _ _ _ _ _ _ _ _ _ _]
      timeout: _ -> [_ _ _ _ _ _ _ _ _ _ _ _ _ _ _ _ _ _ _]
      tunnel: w409 -> [_ _ _ w459 _ w484 w486 _ _ _ _ _ _ _ _ _ _ _ _]
      tunnel: w408 -> [_ _ _ _ _ _ _ _ _ _ _ _ _ w577 _ w597 w606 _ _]
      tunnel: w407 -> [_ _ _ _ _ _ _ _ _ _ _ _ _ w575 _ w595 w608 w616 w623]
      tunnel: w406 -> [_ _ _ _ _ _ _ _ _ _ _ _ _ w576 _ w596 w607 _ _]
      tunnel: w405 -> [_ _ _ _ _ _ _ _ _ _ _ _ _ w571 _ _ _ _ _]
      tunnel: w404 -> [_ _ _ _ _ _ _ _ _ _ _ _ _ _ _ w591 _ _ _]
      tunnel: w403 -> [_ _ _ _ _ _ _ _ _ _ _ _ _ _ _ _ _ w614 _]
      event Timeout {
        n238 = event-data() -> ()  [unwired: 1 in, 3 out]
      }
      event "质控参数设置": Value Change {
        n239 = event-data() -> ()  [unwired: 1 in, 6 out]
        n240 = global read "总磷氨氮断电保存全局变量.vi" "质控参数设置"() -> (w411:T20)
        n241 = call "总磷氨氮质控参数设置.vi"("质控参数设置"=w411) -> ("输出簇"=w412:T21)  [unwired: 10 in]
        n242 = Unbundle By Name(w412) -> ("确定"=w413:bool)
        n243 = case shown="真" w413 {
          tunnel: w412 -> [_ w415]
          tunnel: w411 -> [_ w414]
          frame False {
          }
          frame True {
            n244 = flat-sequence {
              tunnel: w415 -> [w426]
              tunnel: w414 -> [w425]
              frame #0 {
                n245 = Unbundle By Name(w426) -> ("总磷跨度值"=w417:dbl, "总磷零点标准液浓度"=w418:dbl, "总磷跨度标准液浓度"=w419:dbl, "总磷标准液标准浓度"=w420:dbl, "氨氮跨度值"=w421:dbl, "氨氮零点标准液浓度"=w422:dbl, "氨氮跨度标准液浓度"=w423:dbl, "氨氮标准液标准浓度"=w424:dbl)
                n246 = Bundle By Name(cluster=w425, "总磷跨度值"=w417, "总磷零点标准液浓度"=w418, "总磷跨度标准液浓度"=w419, "总磷标准液标准浓度"=w420, "氨氮跨度值"=w421, "氨氮零点标准液浓度"=w422, "氨氮跨度标准液浓度"=w423, "氨氮标准液标准浓度"=w424) -> (w416:T20)
                n247 = global write "总磷氨氮断电保存全局变量.vi" "质控参数设置"(w416) -> ()
              }
              frame #1 {
                n248 = call <vilib>:"Application Directory.vi"() -> ("Application Directory"=w427:path)
                n249 = Build Path(base path=w427, name or relative path="data\\sys.ini" ("名称或相对路径")) -> (appended path=w429:path)
                n250 = call <vilib>:"Open Config Data.vi"("configuration file path"=w429) -> ("error out"=w433:errorcluster, "refnum"=w430:T18)  [unwired: 8 in, 1 out]
                n251 = vi-ref "氨氮总磷.lvlib:总磷氨氮断电保存全局变量.vi"() -> (w431:refnum<vi>)
                n252 = call <userlib>:"Write Panel to INI__ogtk.vi"("error in (no error)"=w433, "VI ref"=w431, "refnum"=w430) -> ("error out"=w434:errorcluster, "refnum out"=w432:T18)  [unwired: 7 in]
                n253 = call <vilib>:"Close Config Data.vi"("error in (no error)"=w434, "refnum"=w432) -> ("error out"=w439:errorcluster, "file path"=w440:path)  [unwired: 8 in]
                n254 = Open/Create/Replace File(file path (use dialog)=w440, error in=w439) -> (refnum out=w436:refnum<file>, error out=w435:errorcluster)  [unwired: 4 in, 1 out]
                n255 = Flush File(refnum=w436, error in=w435) -> (refnum out=w437:refnum<file>, error out=w438:errorcluster)
                n256 = Close File(refnum=w437, error in=w438) -> ()  [unwired: 2 out]
              }
            }
          }
        }
      }
      event "总磷自动测试量程配置", "氨氮自动测试量程配置": Value Change {
        n257 = event-data() -> ()  [unwired: 1 in, 6 out]
        n258 = flat-sequence {
          frame #0 {
            n259 = global write "总磷氨氮断电保存全局变量.vi" "氨氮自动测试量程配置"("氨氮自动测试量程配置") -> ()
            n260 = global write "总磷氨氮断电保存全局变量.vi" "总磷自动测试量程配置"("总磷自动测试量程配置") -> ()
          }
          frame #1 {
            n261 = call <vilib>:"Application Directory.vi"() -> ("Application Directory"=w443:path)
            n262 = Build Path(base path=w443, name or relative path="data\\sys.ini" ("名称或相对路径")) -> (appended path=w445:path)
            n263 = call <vilib>:"Open Config Data.vi"("configuration file path"=w445) -> ("error out"=w449:errorcluster, "refnum"=w446:T18)  [unwired: 8 in, 1 out]
            n264 = vi-ref "氨氮总磷.lvlib:总磷氨氮断电保存全局变量.vi"() -> (w447:refnum<vi>)
            n265 = call <userlib>:"Write Panel to INI__ogtk.vi"("error in (no error)"=w449, "VI ref"=w447, "refnum"=w446) -> ("error out"=w450:errorcluster, "refnum out"=w448:T18)  [unwired: 7 in]
            n266 = call <vilib>:"Close Config Data.vi"("error in (no error)"=w450, "refnum"=w448) -> ("error out"=w455:errorcluster, "file path"=w456:path)  [unwired: 8 in]
            n267 = Open/Create/Replace File(file path (use dialog)=w456, error in=w455) -> (refnum out=w452:refnum<file>, error out=w451:errorcluster)  [unwired: 4 in, 1 out]
            n268 = Flush File(refnum=w452, error in=w451) -> (refnum out=w453:refnum<file>, error out=w454:errorcluster)
            n269 = Close File(refnum=w453, error in=w454) -> ()  [unwired: 2 out]
          }
        }
      }
      event "手动启动": Value Change {
        n270 = event-data() -> ()  [unwired: 1 in, 6 out]
        n271 = call "总磷氨氮启动参数对话框.vi"() -> ("确认"=w457:bool, "元素"=w458:cluster{"命令":string, "data":variant})  [unwired: 10 in]
        n272 = case shown="真" w457 {
          tunnel: w459 -> [_ w461]
          tunnel: w458 -> [_ w460]
          frame False {
          }
          frame True {
            n273 = Enqueue Element(queue=w461, element=w460) -> ()  [unwired: 2 in, 3 out]
          }
        }
      }
      event "定时启动": Mouse Down {
        n274 = event-data() -> ()  [unwired: 1 in, 6 out]
        n275 = flat-sequence {
          frame #0 {
            n276 = global read "总磷氨氮断电保存全局变量.vi" "定时控制"() -> (w463:T7)
            n277 = call "总磷氨氮周期设置.vi"("定时控制参数输入"=w463) -> ("定时控制参数输出"=w462:T7)  [unwired: 10 in]
            n278 = global write "总磷氨氮断电保存全局变量.vi" "定时控制"(w462) -> ()
          }
          frame #1 {
            n279 = call <vilib>:"Application Directory.vi"() -> ("Application Directory"=w464:path)
            n280 = Build Path(base path=w464, name or relative path="data\\sys.ini" ("名称或相对路径")) -> (appended path=w466:path)
            n281 = call <vilib>:"Open Config Data.vi"("configuration file path"=w466) -> ("error out"=w470:errorcluster, "refnum"=w467:T18)  [unwired: 8 in, 1 out]
            n282 = vi-ref "氨氮总磷.lvlib:总磷氨氮断电保存全局变量.vi"() -> (w468:refnum<vi>)
            n283 = call <userlib>:"Write Panel to INI__ogtk.vi"("error in (no error)"=w470, "VI ref"=w468, "refnum"=w467) -> ("error out"=w471:errorcluster, "refnum out"=w469:T18)  [unwired: 7 in]
            n284 = call <vilib>:"Close Config Data.vi"("error in (no error)"=w471, "refnum"=w469) -> ("error out"=w476:errorcluster, "file path"=w477:path)  [unwired: 8 in]
            n285 = Open/Create/Replace File(file path (use dialog)=w477, error in=w476) -> (refnum out=w473:refnum<file>, error out=w472:errorcluster)  [unwired: 4 in, 1 out]
            n286 = Flush File(refnum=w473, error in=w472) -> (refnum out=w474:refnum<file>, error out=w475:errorcluster)
            n287 = Close File(refnum=w474, error in=w475) -> ()  [unwired: 2 out]
          }
        }
      }
      event "单步测试": Value Change {
        w479 = u16 1 items=["总磷"=1, "氨氮"=3] ("站号")
        n288 = event-data() -> ()  [unwired: 1 in, 6 out]
        n289 = Bundle("站号"=w479, "总磷氨氮调试"="总磷氨氮调试") -> (w478:cluster{"站号":u16, "总磷氨氮调试":u16[]})  [unwired: 1 in]
        n290 = Bundle By Name(cluster=cluster{"命令":string, "data":variant} {"命令"="", "data"=variant} ("元素"), "命令"="debug", "data"=w478) -> (w481:cluster{"命令":string, "data":variant})
        n291 = Enqueue Element(queue=w484, element=w481) -> ()  [unwired: 2 in, 3 out]
      }
      event "停止": Value Change {
        n292 = event-data() -> ()  [unwired: 1 in, 6 out]
        n293 = Enqueue Element(queue=w486, element=cluster{"命令":string, "data":variant} {"命令"="启动", "data"=variant(cluster{"站号":u16, "控制命令输出":u16[]} {"站号"=1, "控制命令输出"=[2816]})} ("元素")) -> ()  [unwired: 2 in, 3 out]
      }
      event "设置": Value Change {
        n294 = event-data() -> ()  [unwired: 1 in, 6 out]
        n295 = property on="窗格" class="Pane"("Origin"=T10 {"Horizontal"=0, "Vertical"=628} ("原点")) -> ()  [unwired: 2 in, 2 out]
      }
      event "返回": Value Change {
        n296 = event-data() -> ()  [unwired: 1 in, 6 out]
        n297 = property on="窗格" class="Pane"("Origin"=T10 {"Horizontal"=0, "Vertical"=0} ("原点")) -> ()  [unwired: 2 in, 2 out]
      }
      event "标液浓度1", "测量吸光度1", "测量吸光度2", "标液浓度2", "测量吸光度3", "标液浓度3", "测量吸光度4", "标液浓度4", "测量吸光度5", "标液浓度5", "样品1启用", "样品3启用", "样品4启用", "样品5启用", "样品2启用", "模型", "method", "精度": Value Change {
        n298 = event-data() -> ()  [unwired: 1 in, 6 out]
        n299 = Replace Array Subset(array=dbl[] [0.0, 0.0, 0.0, 0.0, 0.0] ("数组"), new element #1="标液浓度1", new element #2="标液浓度2", new element #3="标液浓度3", new element #4="标液浓度4", new element #5="标液浓度5") -> (w524:dbl[])  [unwired: 5 in]
        n300 = Replace Array Subset(array=dbl[] [0.0, 0.0, 0.0, 0.0, 0.0] ("数组"), new element #1="测量吸光度1", new element #2="测量吸光度2", new element #3="测量吸光度3", new element #4="测量吸光度4", new element #5="测量吸光度5") -> (w523:dbl[])  [unwired: 5 in]
        n301 = Replace Array Subset(array=bool[] [FALSE, FALSE, FALSE, FALSE, FALSE] ("数组"), new element #1="样品1启用", new element #2="样品2启用", new element #3="样品3启用", new element #4="样品4启用", new element #5="样品5启用") -> (w522:bool[])  [unwired: 5 in]
        n302 = call "线性公式.vi"("精度"="精度", "模型"="模型", "method"="method", "启用"=w522, "监测浓度"=w523, "标液浓度"=w524) -> ("XY图"=w499:cluster{"X Values":dbl[], "Y Values":dbl[]}[], "r^2"=w500:dbl, "拟合方程"=w501:string)  [unwired: 3 in]
        "XY图" <- w499
        "拟合公式" <- w501
        "r^2" <- w500
        n303 = global read "总磷氨氮断电保存全局变量.vi" "曲线模型"() -> (w521:T19)
        n304 = local read "样品1 F0"() -> (w498:dbl)
        n305 = local read "样品1 F1"() -> (w497:dbl)
        n306 = local read "样品2 F0"() -> (w496:dbl)
        n307 = local read "样品2 F1"() -> (w495:dbl)
        n308 = local read "样品3 F0"() -> (w494:dbl)
        n309 = local read "样品3 F1"() -> (w493:dbl)
        n310 = local read "样品4 F0"() -> (w492:dbl)
        n311 = local read "样品4 F1"() -> (w491:dbl)
        n312 = local read "样品5 F0"() -> (w490:dbl)
        n313 = local read "样品5 F1"() -> (w489:dbl)
        n314 = Bundle By Name(cluster=w521, "标液浓度1"="标液浓度1", "标液浓度2"="标液浓度2", "标液浓度3"="标液浓度3", "标液浓度4"="标液浓度4", "标液浓度5"="标液浓度5", "测量吸光度1"="测量吸光度1", "测量吸光度2"="测量吸光度2", "测量吸光度3"="测量吸光度3", "测量吸光度4"="测量吸光度4", "测量吸光度5"="测量吸光度5", "样品1启用"="样品1启用", "样品2启用"="样品2启用", "样品3启用"="样品3启用", "样品4启用"="样品4启用", "样品5启用"="样品5启用", "模型"="模型", "method"="method", "精度"="精度", "拟合公式"=w501, "r^2"=w500, "XY图"=w499, "样品1 F0"=w498, "样品1 F1"=w497, "样品2 F0"=w496, "样品2 F1"=w495, "样品3 F0"=w494, "样品3 F1"=w493, "样品4 F0"=w492, "样品4 F1"=w491, "样品5 F0"=w490, "样品5 F1"=w489) -> (w520:T19)
        n315 = flat-sequence {
          tunnel: w520 -> [w528]
          frame #0 {
            n316 = global write "总磷氨氮断电保存全局变量.vi" "曲线模型"(w528) -> ()
          }
          frame #1 {
            n317 = call <vilib>:"Application Directory.vi"() -> ("Application Directory"=w542:path)
            n318 = Build Path(base path=w542, name or relative path="data\\sys.ini" ("名称或相对路径")) -> (appended path=w540:path)
            n319 = call <vilib>:"Open Config Data.vi"("configuration file path"=w540) -> ("error out"=w536:errorcluster, "refnum"=w539:T18)  [unwired: 8 in, 1 out]
            n320 = vi-ref "氨氮总磷.lvlib:总磷氨氮断电保存全局变量.vi"() -> (w538:refnum<vi>)
            n321 = call <userlib>:"Write Panel to INI__ogtk.vi"("error in (no error)"=w536, "VI ref"=w538, "refnum"=w539) -> ("error out"=w535:errorcluster, "refnum out"=w537:T18)  [unwired: 7 in]
            n322 = call <vilib>:"Close Config Data.vi"("error in (no error)"=w535, "refnum"=w537) -> ("error out"=w530:errorcluster, "file path"=w529:path)  [unwired: 8 in]
            n323 = Open/Create/Replace File(file path (use dialog)=w529, error in=w530) -> (refnum out=w533:refnum<file>, error out=w534:errorcluster)  [unwired: 4 in, 1 out]
            n324 = Flush File(refnum=w533, error in=w534) -> (refnum out=w532:refnum<file>, error out=w531:errorcluster)
            n325 = Close File(refnum=w532, error in=w531) -> ()  [unwired: 2 out]
          }
        }
      }
      event "样品1 F0", "样品1 F1", "样品2 F1", "样品2 F0", "样品3 F1", "样品3 F0", "样品4 F0", "样品4 F1", "样品5 F1", "样品5 F0": Value Change {
        n326 = event-data() -> ()  [unwired: 1 in, 6 out]
        n327 = formula code="E=log(F0/F1);"("F0"="样品5 F0", "F1"="样品5 F1") -> ("E"=w543:dbl)
        n328 = formula code="E=log(F0/F1);"("F0"="样品4 F0", "F1"="样品4 F1") -> ("E"=w544:dbl)
        n329 = formula code="E=log(F0/F1);"("F0"="样品3 F0", "F1"="样品3 F1") -> ("E"=w545:dbl)
        n330 = formula code="E=log(F0/F1);"("F0"="样品2 F0", "F1"="样品2 F1") -> ("E"=w546:dbl)
        n331 = formula code="E=log(F0/F1);"("F0"="样品1 F0", "F1"="样品1 F1") -> ("E"=w547:dbl)
        n332 = property on="测量吸光度5" class="DigNum (严格)"("Val(Sgnl)"=w543) -> ()  [unwired: 2 in, 2 out]
        n333 = property on="测量吸光度4" class="DigNum (严格)"("Val(Sgnl)"=w544) -> ()  [unwired: 2 in, 2 out]
        n334 = property on="测量吸光度3" class="DigNum (严格)"("Val(Sgnl)"=w545) -> ()  [unwired: 2 in, 2 out]
        n335 = property on="测量吸光度2" class="DigNum (严格)"("Val(Sgnl)"=w546) -> ()  [unwired: 2 in, 2 out]
        n336 = property on="测量吸光度1" class="DigNum (严格)"("Val(Sgnl)"=w547) -> ()  [unwired: 2 in, 2 out]
      }
      event "标液浓度1", "标液浓度2", "标液浓度3", "标液浓度4", "标液浓度5", "样品1 F0", "样品1 F1", "样品2 F1", "样品2 F0", "样品3 F1", "样品3 F0", "样品4 F0", "样品4 F1", "样品5 F0", "样品5 F1", "精度", "公式.X^2", "公式.X", "公式.b", "量程切换阈值.阈值", "量程切换阈值.标液浓度", "备用系数.量程上限", "备用系数.量程下限", "备用系数.检出限", "备用系数.精度": Mouse Down {
        n337 = event-data() -> ("CtlRef"=w561:refnum<vi>)  [unwired: 1 in, 5 out]
        n338 = property class="DigNum (严格)"(reference=w561) -> (reference out=w559:refnum<vi>, "Value"=w560:dbl)  [unwired: 1 in, 1 out]
        n339 = call "数字键盘.vi"("OldNumber"=w560) -> ("NewNumber"=w558:dbl)
        n340 = property class="DigNum (严格)"(reference=w559, "Val(Sgnl)"=w558) -> ()  [unwired: 1 in, 2 out]
      }
      event "测量吸光度1", "测量吸光度2", "测量吸光度3", "测量吸光度4", "测量吸光度5": Mouse Down {
        n341 = event-data() -> ("CtlRef"=w566:refnum<vi>)  [unwired: 1 in, 5 out]
        n342 = property class="DigNum (严格)"(reference=w566) -> (reference out=w565:refnum<vi>, "Value"=w563:dbl)  [unwired: 1 in, 1 out]
        n343 = call "数字键盘.vi"("OldNumber"=w563) -> ("NewNumber"=w564:dbl)
        n344 = property class="DigNum (严格)"(reference=w565, "Val(Sgnl)"=w564) -> ()  [unwired: 1 in, 2 out]
        n345 = Not Equal?(x=w564, y=w563) -> (x != y?=w562:bool)
        n346 = case shown="真" w562 {
          frame False {
          }
          frame True {
            w567 = 0.0 ("样品1 F0")
            n347 = local write "样品1 F0"(w567) -> ()
            n348 = local write "样品1 F1"(w567) -> ()
            n349 = local write "样品2 F0"(w567) -> ()
            n350 = local write "样品2 F1"(w567) -> ()
            n351 = local write "样品3 F0"(w567) -> ()
            n352 = local write "样品3 F1"(w567) -> ()
            n353 = local write "样品4 F0"(w567) -> ()
            n354 = local write "样品4 F1"(w567) -> ()
            n355 = local write "样品5 F0"(w567) -> ()
            n356 = local write "样品5 F1"(w567) -> ()
          }
        }
      }
      event "读公式": Value Change {
        n357 = event-data() -> ()  [unwired: 1 in, 6 out]
        n358 = property class="Enum (严格)"(reference=w575) -> ("Value"=w574:enum16{"氨氮", "总磷"})  [unwired: 1 in, 2 out]
        n359 = property class="Enum (严格)"(reference=w576) -> ("Value"=w573:enum16{"水样测量", "空白核查", "标样核查", "盲样测试", "加标回收"})  [unwired: 1 in, 2 out]
        n360 = property class="Enum (严格)"(reference=w577) -> ("Value"=w572:enum16{"低量程", "高量程"})  [unwired: 1 in, 2 out]
        n361 = call "总磷氨氮公式读取.vi"("量程"=w572, "测量模式"=w573, "测量参数"=w574) -> ("error out"=w569:errorcluster, "公式"=w570:cluster{"X^2":dbl, "X":dbl, "b":dbl})  [unwired: 7 in]
        n362 = property class="Clust (严格)"(reference=w571, "Value"=w570) -> ()  [unwired: 1 in, 2 out]
        n363 = case shown="错误" w569 {
          tunnel: ["读取成功" ("消息") "读取失败" ("消息")] -> w568
          frame No Error {
          }
          frame Error {
          }
        }
        n364 = One Button Dialog(message=w568) -> ()  [unwired: 1 in, 1 out]
      }
      event "写公式": Value Change {
        n365 = event-data() -> ()  [unwired: 1 in, 6 out]
        n366 = call "总磷氨氮公式写入.vi"("公式"="公式", "量程"="量程下拉列表", "测量模式"="测量模式下拉列表", "测量参数"="参数下拉列表") -> ("error out"=w580:errorcluster)  [unwired: 7 in]
        n367 = case shown="无错误" w580 {
          tunnel: ["写入成功" ("消息") "写入失败" ("消息")] -> w581
          frame No Error {
          }
          frame Error {
          }
        }
        n368 = One Button Dialog(message=w581) -> ()  [unwired: 1 in, 1 out]
      }
      event "量程切换阈值读取": Value Change {
        n369 = event-data() -> ()  [unwired: 1 in, 6 out]
        n370 = property class="Enum (严格)"(reference=w595) -> ("Value"=w594:enum16{"氨氮", "总磷"})  [unwired: 1 in, 2 out]
        n371 = property class="Enum (严格)"(reference=w596) -> ("Value"=w593:enum16{"水样测量", "空白核查", "标样核查", "盲样测试", "加标回收"})  [unwired: 1 in, 2 out]
        n372 = property class="Enum (严格)"(reference=w597) -> ("Value"=w592:enum16{"低量程", "高量程"})  [unwired: 1 in, 2 out]
        n373 = call "总磷氨氮量程读取.vi"("量程"=w592, "测量模式"=w593, "测量参数"=w594) -> ("error out"=w588:errorcluster, "量程切换阈值"=w590:cluster{"阈值":dbl, "标液浓度":dbl})  [unwired: 7 in]
        n374 = property class="Clust (严格)"(reference=w591, "Value"=w590) -> ()  [unwired: 1 in, 2 out]
        n375 = case shown="错误" w588 {
          tunnel: ["读取成功" ("消息") "读取失败" ("消息")] -> w589
          frame No Error {
          }
          frame Error {
          }
        }
        n376 = One Button Dialog(message=w589) -> ()  [unwired: 1 in, 1 out]
      }
      event "量程切换阈值写入": Value Change {
        n377 = event-data() -> ()  [unwired: 1 in, 6 out]
        n378 = property class="Enum (严格)"(reference=w608) -> ("Value"=w605:enum16{"氨氮", "总磷"})  [unwired: 1 in, 2 out]
        n379 = property class="Enum (严格)"(reference=w607) -> ("Value"=w604:enum16{"水样测量", "空白核查", "标样核查", "盲样测试", "加标回收"})  [unwired: 1 in, 2 out]
        n380 = property class="Enum (严格)"(reference=w606) -> ("Value"=w603:enum16{"低量程", "高量程"})  [unwired: 1 in, 2 out]
        n381 = call "总磷氨氮量程写入.vi"("量程切换阈值"="量程切换阈值", "量程"=w603, "测量模式"=w604, "测量参数"=w605) -> ("error out"=w600:errorcluster)  [unwired: 7 in]
        n382 = case shown="无错误" w600 {
          tunnel: ["写入成功" ("消息") "写入失败" ("消息")] -> w601
          frame No Error {
          }
          frame Error {
          }
        }
        n383 = One Button Dialog(message=w601) -> ()  [unwired: 1 in, 1 out]
      }
      event "备用系数读取": Value Change {
        n384 = event-data() -> ()  [unwired: 1 in, 6 out]
        n385 = property class="Enum (严格)"(reference=w616) -> ("Value"=w615:enum16{"氨氮", "总磷"})  [unwired: 1 in, 2 out]
        n386 = call "总磷氨氮备用系数读取.vi"("测量参数"=w615) -> ("error out"=w611:errorcluster, "备用系数"=w613:T3)  [unwired: 9 in]
        n387 = property class="Clust (严格)"(reference=w614, "Value"=w613) -> ()  [unwired: 1 in, 2 out]
        n388 = case shown="错误" w611 {
          tunnel: ["读取成功" ("消息") "读取失败" ("消息")] -> w612
          frame No Error {
          }
          frame Error {
          }
        }
        n389 = One Button Dialog(message=w612) -> ()  [unwired: 1 in, 1 out]
      }
      event "备用系数写入": Value Change {
        n390 = event-data() -> ()  [unwired: 1 in, 6 out]
        n391 = property class="Enum (严格)"(reference=w623) -> ("Value"=w622:enum16{"氨氮", "总磷"})  [unwired: 1 in, 2 out]
        n392 = call "总磷氨氮备用系数写入.vi"("备用系数"="备用系数", "测量参数"=w622) -> ("error out"=w619:errorcluster)  [unwired: 9 in]
        n393 = case shown="无错误" w619 {
          tunnel: ["写入成功" ("消息") "写入失败" ("消息")] -> w620
          frame No Error {
          }
          frame Error {
          }
        }
        n394 = One Button Dialog(message=w620) -> ()  [unwired: 1 in, 1 out]
      }
    }
  }
